vi "WS1050 36 DUT Characterization Ver1.1.vi"() -> ()   [LabVIEW 2012]
uses:
  WS_VCAP Driver 029/Source/WSVCAP Shell/Type Defs/WSVCAP SHL I2C DUT Mask Mode Enum.ctl
  <vilib>/Utility/file.llb/Read From Spreadsheet File (DBL).vi
panel:
  out "VISA resource name out":refnum<visa-resource-name>="GPIB0::3::INSTR"
  out "error out 2":errorcluster={"status"=TRUE, "code"=-63192, "source"="niLvFpga_Open_PXI-7813R.vi"}
  in  "Reg1_Bit Cntrl":string[](array[string])=["01", "02", "04", "08", "10", "20", "40", "80", "03", "06", "0C", "D8", "33", "66", "CC", "07", "0E", "1C", "38", "70", "E0", "0F", "1E", "3C", "78", "F0", "1F", "3E", "7C", "F8", "3F", "7E", "FC", "7F", "FE", "FD", "FB", "F7", "EF", "DF", "BF", "7F", "FC", "F9", "F3", "E7", "CF", "9F", "3F", "F8", "F1", "E3", "C7", "8F", "1F", "F0", "E1", "C3", "87", "0F", "E0", "C1", "83", "07", "C0", "81", "03", "AA", "55", "00"]
  out "date string":string="5/19/2014"
  out "PS1 Out":refnum<visa-resource-name>
  out "Ke2000 Out":refnum<visa-resource-name>="GPIB0::9::INSTR"
  in  "VPI_Cmd":string[](array[string])=["00", "3B", "00"]
  in  "VPI Name":string[](array[string])=["All_Drivers OFF", "All Drivers ON", "All Drivers OFF2"]
  in  "Tab Control":T1(tab)
  in  "No of Cmd":i64=3
  in  "Board#":string="BRD5"
  in  "Serial Number":string[][](table)=[["DUT", "SN"], ["DUT1", "1"], ["DUT2", "2"], ["DUT3", "3"], ["DUT4", "4"], ["DUT5", "5"], ["DUT6", "6"], ["DUT7", "7"], ["DUT8", "8"], ["DUT9", "9"], ["DUT10", "10"], ["DUT11", "11"], ["DUT12", "12"], ["DUT13", "13"], ["DUT14", "14"], ["DUT15", "15"], ["DUT16", "16"], ["DUT17", "17"], ["DUT18", "18"], ["DUT19", "19"], ["DUT20", "20"], ["DUT21", "21"], ["DUT22", "22"], ["DUT23", "23"], ["DUT24", "24"], ["DUT25", "25"], ["DUT26", "26"], ["DUT27", "27"], ["DUT28", "28"], ["DUT29", "29"], ["DUT30", "30"], ["DUT31", "31"], ["DUT32", "32"], ["DUT33", "33"], ["DUT34", "34"], ["DUT35", "35"], ["DUT36", "36"]]
  in  "SPI Clock Rate (Hz)":dbl=5000000.0 caption="Cycle Speed" format="%.1p Hz"
  in  "Wafer#":string="T7-EB"
  in  "File Name":string="CYC_WS1050_T7_EB_65C_40V_25DC_EMPTY_BRD5_141017_1"
  in  "TMN DC\\CAP Data Log File Path":path=path "C:/WS1050 36 DUT Data"
  in  "Test Program":string="WS1050 36 DUT Characterization Ver1.1"
  out "Current Date":string="8/28/2014"
  out "Current Time":string="0950"
  in  "Start Date":string="10/21/2014"
  in  "Start Time":string="1542"
  in  "Comment":string="CYC65C40V"
  in  "OK Button":bool
  in  "Calibration":bool
  in  "Verify CP":bool
  in  "CP Setting":i32(ring) items=["CP OFF", "CP ON", "CP 35V", "CP 40V", "DVA ON", "DVA OFF", "REG1 ON", "REG1 OFF", "REG2 ON", "REG2 OFF", "REG3 ON", "REG3 OFF"]
  in  "Stop Calibration":bool
  in  "Set VDD":dbl=3.7 format="%.3g"
  in  "Command":string[](array[string])=["07020100003B", "070201003B00", "0702013B0000"]
  in  "Clock Rate (Hz)":dbl=1000000.0 caption="Meas Speed" format="%.1p Hz"
  out "AR  Measurent(Hz)":dbl
  in  "PS1 Source":refnum<visa-resource-name>="GPIB0::5::INSTR"
  in  "Ke2000":refnum<visa-resource-name>="GPIB0::9::INSTR"
  in  "Set CP to Meas":i32(ring) items=["CP OFF", "CP 23.75V ", "CP 24.5V", "CP 25.25V", "CP 26V", "CP 26.75V", "CP 27.5V", "CP 28.25V", "CP 29V", "CP 29.75V", "CP 30.5V", "CP 31.25V", "CP 32V", "CP 32.75V", "CP 33.5V", "CP 34.25V", "CP 35V", "CP 35.75V", "CP 36.5V", "CP 37.25V", "CP 38V", "CP 38.75V", "CP 39.5V", "CP 40.25V", "CP 41V", "CP 41.75V", "CP 42.5V", "CP 43.25V", "CP 44V", "CP 50V", "CP 55V"]
  out "Simulate FPGA":bool
  out "Online":bool
  out "AR Cycling(Hz)":dbl=5000000.0
  in  "Ke2400":refnum<visa-resource-name>="GPIB0::3::INSTR"
  in  "Initialize AD7747":bool
  in  "DUT Mask Mode":T2=enum."All"
  in  "RFFE Slave Address":u8=7 caption="Slave Address" format="0x%02x"
  out "Activity Log":string="05/19/2014 -- 12:24:35.853::WSVCAP::APP::Application Started\n05/19/2014 -- 12:24:37.606::WSVCAP::WSVCAP SHL::WR I2C-REG:0x0A;MASK:0xFFFFFFFFFFFF;C1 DATA:22:22:22:22:22:22:22:22:22:22:22:22:22:22:22:22;C2 DATA:22:22:22:22:22:22:22:22:22:22:22:22:22:22:22:22;C3 DATA:22:22:22:22:22:22:22:22:22:22:22:22:22:22:22:22\r\n05/19/2014 -- 12:24:37.773::WSVCAP::WSVCAP SHL::WR I2C-ST:0,0,4,1\r\n05/19/2014 -- 12:24:37.903::WSVCAP::WSVCAP SHL::RD I2C-BYTES:4;ADD:0x00;MASK:0xFFFFFFFFFFFF\r\n05/19/2014 -- 12:24:38.045::WSVCAP::WSVCAP SHL::RD I2C:C1 DATA:2:2:2:2:2:2:2:2:2:2:2:2:2:2:2:2|A7:A9:AA:82:82:7F:82:81:82:81:83:82:81:82:82:81|46:36:BB:88:44:A3:E9:2B:32:20:ED:25:BB:3D:68:B|2C:6A:EB:A7:22:56:FE:CC:36:82:D7:B0:3B:48:F9:CC;C2 DATA:2:2:2:2:2:2:2:2:2:2:2:2:2:2:2:2|94:94:94:80:80:80:80:80:81:7E:7E:81:80:7E:80:80|47:33:15:82:62:B:E8:1C:D7:C3:7D:41:7C:B7:4C:2A|C4:B4:AE:8:1E:D1:4E:37:11:C0:6F:63:42:9D:63:B5;C3 DATA:2:2:2:2:2:2:2:2:2:2:2:2:2:2:2:2|95:95:95:81:81:7E:81:80:84:7D:80:83:81:7E:7F:80|AB:C4:14:B5:7B:52:DF:C9:79:5D:5F:30:99:31:1E:F4|6E:5C:F7:A8:C3:EB:7B:EF:33:92:89:77:4D:67:75:DD;STATUS:0:0:4:0\r\n05/19/2014 -- 12:24:38.046::WSVCAP::WSVCAP SHL::WR I2C-REG:0x0A;MASK:0xFFFFFFFFFFFF;C1 DATA:22:22:22:22:22:22:22:22:22:22:22:22:22:22:22:22;C2 DATA:22:22:22:22:22:22:22:22:22:22:22:22:22:22:22:22;C3 DATA:22:22:22:22:22:22:22:22:22:22:22:22:22:22:22:22\r\n05/19/2014 -- 12:24:38.089::WSVCAP::WSVCAP SHL::WR I2C-ST:0,0,4,1\r\n05/19/2014 -- 12:24:38.219::WSVCAP::WSVCAP SHL::RD I2C-BYTES:4;ADD:0x00;MASK:0xFFFFFFFFFFFF\r\n05/19/2014 -- 12:24:38.362::WSVCAP::WSVCAP SHL::RD I2C:C1 DATA:2:2:2:2:2:2:2:2:2:2:2:2:2:2:2:2|A7:AB:AA:82:82:82:83:83:82:82:82:82:7F:82:82:81|4B:32:96:83:3E:61:43:17:25:62:AB:4D:A2:40:2E:5|3C:76:2B:B4:EE:E4:A9:1A:AA:A:26:C7:21:2E:87:5B;C2 DATA:2:2:2:2:2:2:2:2:2:2:2:2:2:2:2:2|94:94:94:80:80:80:80:80:80:7F:80:81:80:80:7F:80|4A:32:19:7D:19:6C:79:46:61:7F:4B:B8:A5:30:F3:14|B4:70:A:8C:9C:DC:43:FA:1E:A:C6:21:A:A9:13:F3;C3 DATA:2:2:2:2:2:2:2:2:2:2:2:2:2:2:2:2|95:97:94:81:80:81:82:81:80:7E:81:84:7F:81:80:80|B2:32:D0:A7:9E:4C:AB:D4:EE:D9:F0:82:B7:91:7:FF|C1:91:B6:3D:D8:E:1B:4F:9F:6A:F1:6C:E7:3F:7:BA;STATUS:0:0:4:0\r\n05/19/2014 -- 12:24:38.364::WSVCAP::WSVCAP SHL::WR I2C-REG:0x0A;MASK:0xFFFFFFFFFFFF;C1 DATA:22:22:22:22:22:22:22:22:22:22:22:22:22:22:22:22;C2 DATA:22:22:22:22:22:22:22:22:22:22:22:22:22:22:22:22;C3 DATA:22:22:22:22:22:22:22:22:22:22:22:22:22:22:22:22\r\n05/19/2014 -- 12:24:38.406::WSVCAP::WSVCAP SHL::WR I2C-ST:0,0,4,1\r\n05/19/2014 -- 12:24:38.536::WSVCAP::WSVCAP SHL::RD I2C-BYTES:4;ADD:0x00;MASK:0xFFFFFFFFFFFF\r\n05/19/2014 -- 12:24:38.678::WSVCAP::WSVCAP SHL::RD I2C:C1 DATA:2:2:2:2:2:2:2:2:2:2:2:2:2:2:2:2|A7:A9:AB:82:82:81:82:82:82:82:82:82:82:82:82:81|46:71:4C:87:43:3D:7F:FC:25:4F:8E:54:97:3E:60:8C|AA:F4:1F:B5:CE:43:1F:36:9:87:9C:78:86:5:B6:8E;C2 DATA:2:2:2:2:2:2:2:2:2:2:2:2:2:2:2:2|94:94:94:80:7F:7F:80:80:80:80:80:81:80:80:80:80|49:36:18:7D:6E:C5:E4:3C:81:2E:41:D3:75:71:E3:72|E8:D3:E6:D1:E0:48:AE:D4:54:D:E8:8E:B4:41:68:4;C3 DATA:2:2:2:2:2:2:2:2:2:2:2:2:2:2:2:2|95:95:95:81:7F:7F:81:81:81:81:81:84:81:81:82:81|B3:F5:90:AB:82:69:7B:93:D0:77:E8:D5:E8:8C:84:E8|B9:AC:EE:2B:B6:71:8F:4A:74:31:56:BB:8A:B7:A0:C8;STATUS:0:0:4:0\r\n05/19/2014 -- 12:24:38.681::WSVCAP::WSVCAP SHL::WR I2C-REG:0x0A;MASK:0xFFFFFFFFFFFF;C1 DATA:22:22:22:22:22:22:22:22:22:22:22:22:22:22:22:22;C2 DATA:22:22:22:22:22:22:22:22:22:22:22:22:22:22:22:22;C3 DATA:22:22:22:22:22:22:22:22:22:22:22:22:22:22:22:22\r\n05/19/2014 -- 12:24:38.723::WSVCAP::WSVCAP SHL::WR I2C-ST:0,0,4,1\r\n05/19/2014 -- 12:24:38.854::WSVCAP::WSVCAP SHL::RD I2C-BYTES:4;ADD:0x00;MASK:0xFFFFFFFFFFFF\r\n05/19/2014 -- 12:24:38.996::WSVCAP::WSVCAP SHL::RD I2C:C1 DATA:2:2:2:2:2:2:2:2:2:2:2:2:2:2:2:2|A7:A9:AA:82:82:7F:83:81:82:81:84:82:7F:82:7F:82|43:FB:E:7F:3C:AD:35:35:26:A2:6C:21:4B:3D:8:6|63:9A:E1:F3:95:32:91:42:90:3C:78:1F:5C:D7:5F:D8;C2 DATA:2:2:2:2:2:2:2:2:2:2:2:2:2:2:2:2|94:94:94:80:80:80:80:80:81:80:7E:81:80:7E:7F:80|48:36:18:7F:5E:3D:69:83:DE:AE:A1:9E:31:AE:BB:96|15:A0:44:17:13:FD:CC:C8:6D:B2:EF:A7:C:C7:3B:F;C3 DATA:2:2:2:2:2:2:2:2:2:2:2:2:2:2:2:2|95:96:94:81:81:7E:82:80:84:80:80:84:7F:7E:7D:82|AD:3B:6D:A9:7C:57:9D:F5:7A:96:23:5C:36:2D:ED:5A|CD:46:DB:3B:C7:BD:70:60:33:B8:B:F7:63:A:51:4D;STATUS:0:0:4:0\r\n05/19/2014 -- 12:24:38.998::WSVCAP::WSVCAP SHL::WR I2C-REG:0x0A;MASK:0xFFFFFFFFFFFF;C1 DATA:22:22:22:22:22:22:22:22:22:22:22:22:22:22:22:22;C2 DATA:22:22:22:22:22:22:22:22:22:22:22:22:22:22:22:22;C3 DATA:22:22:22:22:22:22:22:22:22:22:22:22:22:22:22:22\r\n05/19/2014 -- 12:24:39.040::WSVCAP::WSVCAP SHL::WR I2C-ST:0,0,4,1\r\n05/19/2014 -- 12:24:39.170::WSVCAP::WSVCAP SHL::RD I2C-BYTES:4;ADD:0x00;MASK:0xFFFFFFFFFFFF\r\n05/19/2014 -- 12:24:39.311::WSVCAP::WSVCAP SHL::RD I2C:C1 DATA:2:2:2:2:2:2:2:2:2:2:2:2:2:2:2:2|A7:AA:AB:82:82:81:82:81:82:81:82:82:82:82:7F:82|44:F1:90:87:45:44:C8:2C:2C:F1:FC:1B:94:3B:3C:75|4A:49:95:19:99:73:64:3:23:24:F3:A2:5E:7F:C4:B6;C2 DATA:2:2:2:2:2:2:2:2:2:2:2:2:2:2:2:2|94:94:94:80:80:80:80:7F:80:80:7E:80:80:7E:7F:80|4C:36:17:7D:A8:9F:DE:C7:53:6D:8A:F4:41:A5:C6:E0|90:2E:24:C:D9:22:E4:76:3B:40:1D:53:33:B1:3E:4D;C3 DATA:2:2:2:2:2:2:2:2:2:2:2:2:2:2:2:2|95:97:95:81:81:7F:81:80:80:81:7F:82:81:7E:7D:82|AE:2B:A7:AB:CC:CD:A4:38:FD:17:80:F2:92:2D:45:C4|76:E5:D:B9:AD:B5:BA:8D:28:32:9E:42:B7:20:4A:D9;STATUS:0:0:4:0\r\n05/19/2014 -- 12:24:39.313::WSVCAP::WSVCAP SHL::WR I2C-REG:0x0A;MASK:0xFFFFFFFFFFFF;C1 DATA:22:22:22:22:22:22:22:22:22:22:22:22:22:22:22:22;C2 DATA:22:22:22:22:22:22:22:22:22:22:22:22:22:22:22:22;C3 DATA:22:22:22:22:22:22:22:22:22:22:22:22:22:22:22:22\r\n05/19/2014 -- 12:24:39.355::WSVCAP::WSVCAP SHL::WR I2C-ST:0,0,4,1\r\n05/19/2014 -- 12:24:39.486::WSVCAP::WSVCAP SHL::RD I2C-BYTES:4;ADD:0x00;MASK:0xFFFFFFFFFFFF\r\n05/19/2014 -- 12:24:39.628::WSVCAP::WSVCAP SHL::RD I2C:C1 DATA:2:2:2:2:2:2:2:2:2:2:2:2:2:2:2:2|A7:A9:AA:82:82:82:83:82:82:82:82:82:7F:82:7F:82|47:18:E4:87:3E:E7:6:65:25:92:37:38:A8:3E:89:85|7C:A7:7:2B:A3:7A:EC:EF:89:ED:F4:D3:D8:BC:3A:F5;C2 DATA:2:2:2:2:2:2:2:2:2:2:2:2:2:2:2:2|94:94:94:80:7F:80:80:7F:81:80:7E:80:80:80:81:80|49:37:17:80:76:25:6A:F8:DF:55:97:4D:B8:5B:2B:B1|13:E3:9A:3E:1A:2D:4F:B6:DB:E9:61:FA:8B:D6:9:CC;C3 DATA:2:2:2:2:2:2:2:2:2:2:2:2:2:2:2:2|95:95:95:81:7F:80:82:81:84:80:7F:81:80:81:7F:82|AF:93:3B:AF:5B:11:82:E4:7E:C3:2D:72:9:96:D9:A|DB:96:F2:10:5F:64:9A:C6:98:12:27:7D:10:D3:20:D9;STATUS:0:0:4:0\r\n05/19/2014 -- 12:24:40.132::WSVCAP::WSVCAP SHL::CLOSE\r\n"
  in  "C1 Cap DAC":u8=128 caption="B Data In" format="0x%02x"
  in  "C2 Cap DAC":u8=128 caption="B Data In" format="0x%02x"
  in  "C3 Cap DAC":u8=128 caption="B Data In" format="0x%02x"
  out "IDD Brd(uA)":string
  in  "CP to Meas":i32(ring)=1 items=["CP HDC 35V", "CP HDC 40.25V", "CP HDC 27.5V", "CP HDC 30.5V", "CP HDC 44V"]
  in  "CP VPI":i32(ring) items=["CP HDC 35V", "CP HDC 40.25V", "CP HDC 27.5V", "CP HDC 30.5V", "CP HDC 44V"]
  in  "Repeat Meas(s)":u32
  in  "Real No. From\nLookup Table":bool
  in  "Control Panel":T3={"CP C-V \nSweep"=TRUE, "HD/CYC"=FALSE, "E-CAL"=FALSE, "DVA"=FALSE, "VPI"=FALSE, "VSA"=FALSE, "HS"=FALSE}
  out "CP C-V Sweep":bool
  out "HD/CYC":bool
  out "E-CAL":bool
  out "DVA":bool
  out "VPI":bool
  out "VSA":bool
  out "HS":bool
  in  "Lot#":string="WS1050"
  out "AD7747 Values":string[][](table)
  in  "Freq(Hz)":string="12K"
  in  "Reset P/S":bool
  in  "Test Sequences":i32(ring) items=["C1_C2_C3", "C2_C1_C3", "C3_C2_C1"]
  in  "WS1050/51":bool=TRUE
  in  "CP with DVA ON":i32(ring) items=["CP HDC 35V", "CP HDC 40.25V", "CP HDC 27.5V", "CP HDC 30.5V", "CP HDC 44V"]
  in  "% Duty Cycle":string="NA"
  in  "Cmd To HD":string="0702013B3B3B"
  in  "Post CMd Delay":dbl[](array[numeric])=[1.8e-05, 1.8e-05, 1.8e-05] min=0.0 max=0.5 format="%#.0p s"
  in  "Cmin/Act":bool=TRUE
  out "40V_1":string[][](table)
  out "NOM IDD OFF(uA)":string
  out "40V_2":string[][](table)
  out "40V_3":string[][](table)
  out "Total Time":u64
  in  "Set HD/Cycle \nto Complete":u64=50000000000
  out "No of HD/Cycle\nCompleted":u64
  out "Cycle Count":u64 min=1 max=4 step=1
  out "Loop \ncompleted":i32=1
  out "Previous Time":string="12:20:26 PM"
  out "STATUS":string="Idle...."
  out "Total Delta C2(pF)":string[](array[string])
  out "Total Delta C1(pF)":string[](array[string])
  out "Total Delta C3(pF)":string[](array[string])
  out "RB Reg for HD":string[](array[string])
  out "RB Reg for HD/Cycle":string[](array[string])
  out "VPI C2":string[][](table)
  out "VPI C3":string[][](table)
  out "NOM IDD ON (uA)":string
  out "IDD_HD/CYC (uA)":string="164.601255E+0"
  in  "stop During HD/Cycles":bool
  in  "stop":bool
  out "IDD Stdby(uA)":string="2.606990E+0"
  out "VPI C1":string[][](table)
  out "Loops Run":u64
  out "CP Voltage":string
  out "VSA_V1":string[][](table)
  out "VSA_V2":string[][](table)
  out "VSA_V3":string[][](table)
  in  "VSA Voltage(V)":dbl[](array[numeric])=[-10.0, 0.0, 10.0]
  in  "DC_Temp":i32=25
  in  "HD/CYC Temp":i32=25
  in  "Time All ON (s)":u32=120
  in  "Time All OFF (s)":u32=120
  in  "HD_DC (Min)":u64=259200
  out "LPs Count":i32
  in  "X Repeat":i32=100
  out "No LPs to RP":i32
  out "Run Loops":i32=1
  out "TTCompleted":u64=2000
  in  "TTF Completed":u64=50000000000
  out "% Delta C_T0":string[][](array[string])
  out "% Delta C":string[][](array[string])
  out "EFuse RB T0":string[](array[string])
  out "Current EFuse Read back":string[](array[string])
  out "EFuse Readback Status":bool[](array[boolean])
  in  "DeltaC Target Setting(pF)":dbl=7.375
  out "error out":errorcluster
  in  "error in (no error)":errorcluster
  in  "HD RP":dbl=60.0
  in  "Cycle RP":dbl=10000.0
  out "Plot_1":dbl[][](graph) caption="(Y) Multi Plot 2"
  out "Plot_2":dbl[][](graph) caption="(Y) Multi Plot 2"
  out "Plot_3":dbl[][](graph) caption="(Y) Multi Plot 2"
  in  "Debug":bool
  in  "No of Rows\nFrom Spread Sheet":i32
  in  "Plot Delta Cmin":bool=TRUE
  in  "Plot":T4(ring)
  in  "Bank 2":i32(ring)=4 items=["C1", "C2", "C3", "D_C1", "D_C2", "D_C3"]
  in  "Bank":i32(ring)=3 items=["C1", "C2", "C3", "D_C1", "D_C2", "D_C3"]
  in  "Bank 3":i32(ring)=5 items=["C1", "C2", "C3", "D_C1", "D_C2", "D_C3"]
  # "Company:  WiSpry Inc\n20 Fairbanks Ste 198 Irvine CA 92618\n\nAuthor:  Andy V Tran\nCreated:  07/15/2015\nLabVIEW 2012 Pro\nTest Program:  WS1050 36 DUT Characterization Ver1.1\nFPGA: WS_VCAP Driver 029"
  # "Note for HD Duty Cycle:\n1.  Set time to start HD_DC (Min), default is 259200 (6 months) \n2.  Set Time for Duty Cycle ON/OFF, default setting is 2 minutes\n3.  No of Loops to RP = 3600s/(Time ALL ON(s) + Time ALL + OFF(s))\n4.  Set X Repeat = no of runs, default is 100 runs\n5.  Set TTF Completed to stop the test.\n\nVer 1.1 updated based on Ver1.0:\n1.  Updated the control panel ( CP C-V Sweep was set \"Yes\" by default)\n2.  CP Voltage sweep should be set up from look up table."
  # "Minutes"
  # "X1000"
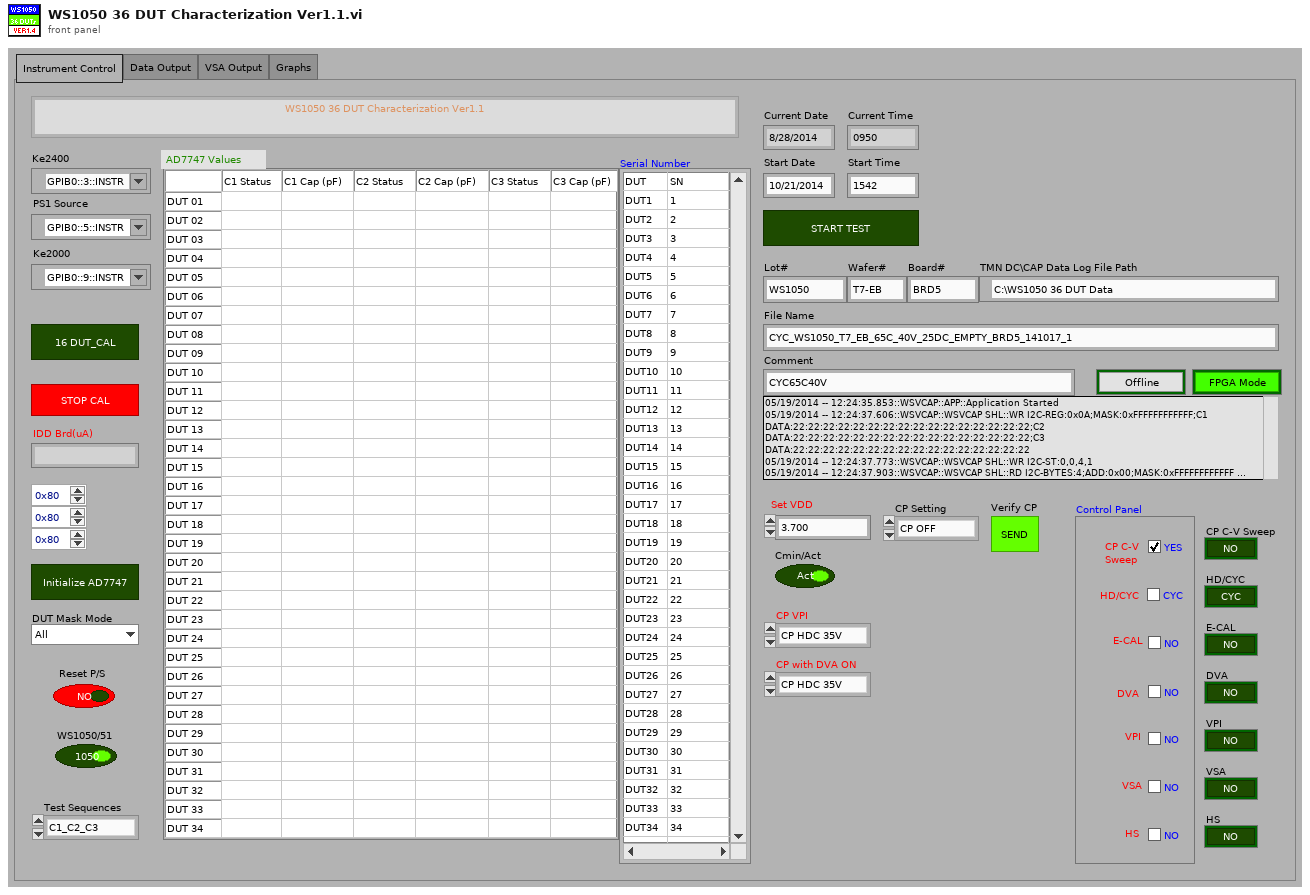
[diagram p1: front panel]
types:
  T1 = enum32{"Instrument Control", "Data Output", "VSA Output", "Graphs"}
  T2 = typedef "WSVCAP SHL I2C DUT Mask Mode Enum.ctl" = enum16{"Custom", "C1", "C2", "C3", "All"}
  T3 = cluster{"CP C-V \nSweep":bool, "HD/CYC":bool, "E-CAL":bool, "DVA":bool, "VPI":bool, "VSA":bool, "HS":bool}
  T4 = enum16{"ALL DUTs", "DUT 01", "DUT 02", "DUT 03", "DUT 04", "DUT 05", "DUT 06", "DUT 07", "DUT 08", "DUT 09", "DUT 10", "DUT 11", "DUT 12", "DUT 13", "DUT 14", "DUT 15", "DUT 16", "DUT 17", "DUT 18", "DUT 19", "DUT 20", "DUT 21", "DUT 22", "DUT 23", "DUT 24", "DUT 25", "DUT 26", "DUT 27", "DUT 28", "DUT 29", "DUT 30", "DUT 31", "DUT 32", "DUT 33", "DUT 34", "DUT 35", "DUT 36"}
  T5 = typedef "WSVCAP SHL Core System Cluster.ctl" = cluster{"Settings":T6, "FPGA Resource":tag, "Online":bool, "I2C Wait Ticks":u32, "SPI Wait Ticks":u32, "RFFE Wait Ticks":u32}
  T6 = typedef "WSVCAP SHL I2C Settings Cluster.ctl" = cluster{"FPGA Resource Name":string, "I2C Slave Address":u8, "I2C Clock Rate (Hz)":dbl, "SPI Clock Rate (Hz)":dbl, "RFFE Slave Address":u8, "RFFE Clock Rate (Hz)":dbl, "Simulate FPGA":bool, "C1 Cap DAC Default":u8, "C2 Cap DAC Default":u8, "C3 Cap DAC Default":u8}
  T7 = enum16{"Idle...", "Voltage 1", "Voltage 2", "Voltage 3"}[]
  T8 = cluster{"Test Program ":string, "Comment":string, "Data Out":string, "Data Out":string, "CP Voltage":string, string, "Data Out":string, "CP Voltage":string, "string":string, "Freq(Hz)":string, "Board#":string}
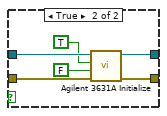
[diagram p2: hidden frame]
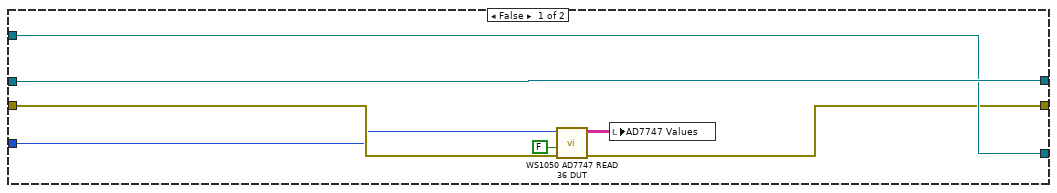
[diagram p10: hidden frame]
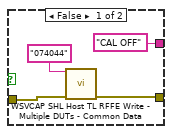
[diagram p11: hidden frame]
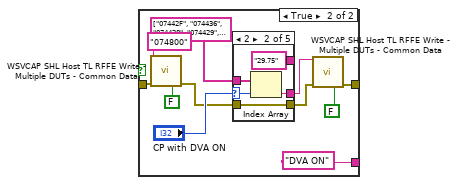
[diagram p12: hidden frame]
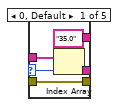
[diagram p13: hidden frame]
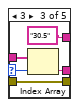
[diagram p14: hidden frame]
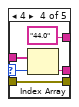
[diagram p15: hidden frame]
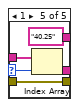
[diagram p16: hidden frame]
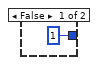
[diagram p17: hidden frame]
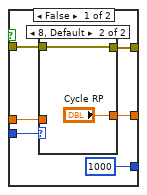
[diagram p18: hidden frame]
diagram:
  w19 = TRUE
  w25 = u16 0 items=["Off", "Moving Filter", "Repeating Filter"] ("Digital Filter (0: Off)")
  w26 = u16 7 items=["3.5 Digits"=4, "4.5 Digits"=5, "5.5 Digits"=6, "6.5 Digits"=7] ("Resolution (7: 6.5 digits)")
  n1 = case shown="True" w19 {
    tunnel: "error in (no error)" -> [w33 w34]
    tunnel: [w33 w41] -> w5
    frame False {
    }
    frame True {
      n2 = call "WSVCAP SHL Host TL Initialize.vi"("error in"=w34) -> ("error out"=w35:errorcluster)  [unwired: 13 in, 1 out]
      n3 = control-ref of="Activity Log"() -> (w37:refnum<vi>)
      n4 = call "ACT LG Activity Log Core.vi"("Display Ref"=w37, "Source"="WSVCAP", "Error In (no error)"=w35) -> ("Error Out"=w36:errorcluster)  [unwired: 11 in, 1 out]
      n5 = call "WSVCAP SHL Host TL Status Manager.vi"("error in"=w36) -> ("System Out"=w42:T5, "error out"=w41:errorcluster)  [unwired: 13 in]
      n6 = Unbundle By Name(w42) -> ("Online"=→"Online":bool, "Settings.Simulate FPGA"=→"Simulate FPGA":bool)
    }
  }
  n7 = case shown="True" TRUE {
    tunnel: w5 -> [w43 w48]
    tunnel: [w44 w47] -> w16
    tunnel: [w43 w46] -> w9
    tunnel: "Ke2400" -> [w44 w45]
    frame False {
    }
    frame True {
      n8 = VISA Write(VISA resource name=w45, write buffer="SOUR:FUNC VOLT;VOLT:MODE FIX;RANG 100;LEV 0.0;:SENS:FUNC \"CURR\";CURR:PROT 60E-3;RANG 100E-3;:OUTP ON", error in (no error)=w48) -> (VISA resource name out=w47:refnum<visa-resource-name>, error out=w46:errorcluster)  [unwired: 1 out]
    }
  }
  n9 = case shown="False" "Reset P/S" {
    tunnel: "PS1 Source" -> [w50 w57]
    tunnel: [w50 w55] -> w30
    tunnel: w5 -> [w51 w53]
    tunnel: [w51 w52] -> w4
    frame False {
    }
    frame True {
      n10 = call "Agilent 3631A Initialize.vi"("error in (no error)"=w53, "Default"=FALSE ("Reset? (T: Yes)"), "Reset"=TRUE ("ID Query? (T: Yes)"), "VISA resource name"=w57) -> ("error out"=w52:errorcluster, "VISA resource name out"=w55:refnum<visa-resource-name>)  [unwired: 6 in]
    }
  }
  n11 = call "Ke2000 Initialize.vi"("error in (no error)"=w5, "VISA resource name"="Ke2000") -> ("error out"=w27:errorcluster, "VISA resource name out"=w28:refnum<visa-resource-name>)  [unwired: 8 in]
  n12 = call "Ke2000 Configure DC Current.vi"("Resolution (7: 6.5 digits)"=w26, "Digital Filter (0: Off)"=w25, "Auto Range? (T: Auto)"=FALSE, "error in (no error)"=w27, "Custom Range (0 A)"=1.0, "VISA resource name"=w28) -> ("error out"=w6:errorcluster, "VISA resource name out"=w23:refnum<visa-resource-name>)  [unwired: 4 in]
  n13 = case shown="True" TRUE {
    tunnel: [_ w58] -> w32
    frame False {
    }
    frame True {
      n14 = call-poly <vilib>:"Read From Spreadsheet File.vi"("number of rows (all:-1)"=-1) -> ("all rows"=w58:dbl[][])  [unwired: 6 in, 4 out]
    }
  }
  n15 = Merge Errors(w9, w6, w4) -> (w17:errorcluster)
  n16 = while {
    tunnel: w17 -> [w62]
    tunnel: [w71] -> w13
    tunnel: w32 -> [w87]
    tunnel: w30 -> [w75]
    tunnel: w23 -> [w76]
    tunnel: [w85] -> w22
    tunnel: [w84] -> w21
    tunnel: w16 -> [w82]
    tunnel: [w81] -> w14
    tunnel: [FALSE ("stop")] -> w7
    i -> [w83]
    stop <- w88 stop-if-true
    n17 = case shown="0" w83 {
      tunnel: w62 -> [w99 w101]
      tunnel: [w98 w101] -> w78
      tunnel: "RFFE Slave Address" -> [w96 _]
      frame 0 {
        w92 = dbl[][] []
        w91 = "" ("uA")
        w93 = string[][] []
        w94 = string[] [] ("EFuse Read back")
        w100 = u64 0 ("No of HD/Cycle\nCompleted")
        n18 = local write "RB Reg for HD/Cycle"(w94) -> ()
        n19 = local write "Current EFuse Read back"(w94) -> ()
        n20 = local write "EFuse RB T0"(w94) -> ()
        n21 = local write "Total Delta C1(pF)"(w94) -> ()
        n22 = local write "Total Delta C2(pF)"(w94) -> ()
        n23 = local write "Total Delta C3(pF)"(w94) -> ()
        n24 = local write "Cycle Count"(w100) -> ()
        n25 = local write "No of HD/Cycle\nCompleted"(w100) -> ()
        n26 = local write "NOM IDD OFF(uA)"(w91) -> ()
        n27 = local write "NOM IDD ON (uA)"(w91) -> ()
        n28 = local write "IDD Brd(uA)"(w91) -> ()
        n29 = local write "40V_2"(w93) -> ()
        n30 = local write "VPI C2"(w93) -> ()
        n31 = local write "VSA_V2"(w93) -> ()
        n32 = local write "VPI C1"(w93) -> ()
        n33 = local write "VPI C3"(w93) -> ()
        n34 = local write "% Delta C_T0"(w93) -> ()
        n35 = local write "40V_1"(w93) -> ()
        n36 = local write "VSA_V3"(w93) -> ()
        n37 = local write "40V_3"(w93) -> ()
        n38 = local write "VSA_V1"(w93) -> ()
        n39 = local write "% Delta C"(w93) -> ()
        n40 = call "WSVCAP SHL Host TL RFFE Configure.vi"("RFFE Slave Address"=w96, "Clock Rate (Hz)"="Clock Rate (Hz)", "error in"=w99) -> ("Actual Rate (Hz)"=→"AR  Measurent(Hz)":dbl, "error out"=w98:errorcluster)  [unwired: 11 in]
        n41 = local write "Plot_3"(w92) -> ()
        n42 = local write "Plot_2"(w92) -> ()
        n43 = local write "Plot_1"(w92) -> ()
      }
      frame 1, Default {
      }
    }
    n44 = while {
      tunnel: ["stop"] -> w80
      tunnel: w78 -> [w127]
      tunnel: [w119] -> w72
      tunnel: w75 -> [w126]
      tunnel: w76 -> [w121]
      tunnel: [w122] -> w74
      tunnel: [w120] -> w73
      tunnel: [w117] -> w69
      tunnel: [w116] -> w68
      tunnel: [w115] -> w67
      tunnel: [w114] -> w66
      tunnel: [w113] -> w65
      tunnel: [w112] -> w64
      tunnel: [w111] -> w63
      tunnel: ["Command"] -> w61
      tunnel: ["Post CMd Delay"] -> w60
      stop <- w134 stop-if-true
      # "Set Date & Time to Start Test"
      n45 = case shown="True" "Initialize AD7747" {
        tunnel: w127 -> [w143 w148]
        tunnel: [w143 w144] -> w110
        tunnel: w126 -> [w142 w146]
        tunnel: [w142 w145] -> w125
        frame False {
        }
        frame True {
          w149 = T7 [enum."Voltage 2", enum."Voltage 3", enum."Voltage 1"] items=["Idle...", "Voltage 1", "Voltage 2", "Voltage 3"]
          n46 = for {
            tunnel: w146 -> [w159]
            tunnel: w149 -> [w157] mode=indexing
            tunnel: [w156] -> w145
            shift-right: [w152] -> w147
            shift-left: w148 -> [w160]
            n47 = local read "Set VDD"() -> (w155:dbl)
            n48 = call "E3631A_Voltage Controller updated.vi"("VISA resource name"=w159, "I_VDD(A)"=0.5, "Channel Controller"=w157, "Voltage 1"=w155, "Voltage 2"=3.3, "error in (no error)"=w160, "I_3.3V (A)"=0.5) -> ("VISA resource name out"=w156:refnum<visa-resource-name>, "error out"=w151:errorcluster)  [unwired: 7 in]
            n49 = call "Delay T4.vi"("milliseconds to wait"=u32 100, "error in (no error)"=w151) -> ("error out"=w152:errorcluster)  [unwired: 9 in]
          }
          n50 = call "WS1050_AD7747_Init 36DUT.vi"("error in"=w147) -> ("error out"=w144:errorcluster)  [unwired: 10 in]
        }
      }
      n51 = call "Time_stamp.vi"() -> ("date/time string"=w139:string, "date string"=w141:string)  [unwired: 2 in]
      "Current Date" <- w141
      "Current Time" <- w139
      n52 = Equal?(x=w141, y="Start Date") -> (x = y?=w137:bool)
      n53 = Equal?(x=w139, y="Start Time") -> (x = y?=w136:bool)
      n54 = And(x=w137, y=w136) -> (x .and. y?=w133:bool)
      n55 = Compound Arithmetic op=OR(w133, "OK Button", "stop") -> (w134:bool)
      n56 = case shown="True" "Calibration" {
        tunnel: w110 -> [w190 w204]
        tunnel: [w184 w201] -> w108
        tunnel: w125 -> [w189 w200]
        tunnel: "DUT Mask Mode" -> [w188 w196]
        tunnel: [w189 w195] -> w123
        tunnel: w121 -> [w187 w194]
        tunnel: [w187 w191] -> w120
        frame False {
          n57 = call "WS1050 AD7747 READ 36 DUT.vi"("error in"=w190, "Log (T)"=FALSE, "DUT Mask Mode (All)"=w188) -> ("error out"=w184:errorcluster, "AD7747 Values"=w185:string[][])  [unwired: 7 in]
          n58 = local write "AD7747 Values"(w185) -> ()
        }
        frame True {
          n59 = flat-sequence {
            tunnel: w204 -> [w213]
            tunnel: [w208] -> w203
            tunnel: w200 -> [w212]
            tunnel: [w211] -> w199
            tunnel: w196 -> [w210]
            tunnel: [w210] -> w197
            tunnel: w194 -> [w206]
            tunnel: [w205] -> w193
            tunnel: w203 -> [w236]
            tunnel: [w235] -> w202
            tunnel: w199 -> [w234]
            tunnel: [w234] -> w198
            tunnel: w197 -> [w233]
            tunnel: w193 -> [w229]
            tunnel: [w229] -> w192
            tunnel: w202 -> [w245]
            tunnel: [w248] -> w201
            tunnel: w198 -> [w247]
            tunnel: [w244] -> w195
            tunnel: w192 -> [w243]
            tunnel: [w243] -> w191
            frame #0 {
              w214 = T7 [enum."Voltage 2", enum."Voltage 3", enum."Voltage 1"] items=["Idle...", "Voltage 1", "Voltage 2", "Voltage 3"]
              n60 = for {
                tunnel: w212 -> [w224]
                tunnel: w214 -> [w222] mode=indexing
                tunnel: [w221] -> w211
                shift-right: [w219] -> w207
                shift-left: w213 -> [w225]
                w216 = 0.5 ("I_VDD(A)")
                n61 = local read "Set VDD"() -> (w217:dbl)
                n62 = call "E3631A_Voltage Controller updated.vi"("VISA resource name"=w224, "I_VDD(A)"=w216, "Channel Controller"=w222, "Voltage 1"=w217, "Voltage 2"=3.3, "error in (no error)"=w225, "I_3.3V (A)"=w216) -> ("VISA resource name out"=w221:refnum<visa-resource-name>, "error out"=w218:errorcluster)  [unwired: 7 in]
                n63 = call "Delay T4.vi"("milliseconds to wait"=u32 100, "error in (no error)"=w218) -> ("error out"=w219:errorcluster)  [unwired: 9 in]
              }
              n64 = call "Ke2000 Single Reading.vi"("error in (no error)"=w207, "VISA resource name"=w206) -> ("error out"=w208:errorcluster, "VISA resource name out"=w205:refnum<visa-resource-name>, "uA"=→"IDD Brd(uA)":string)  [unwired: 5 in, 2 out]
              n65 = One Button Dialog(message="Please verify all sockets should be empty...") -> ()  [unwired: 1 in, 1 out]
            }
            frame #1 {
              n66 = call "WS1050 CAPDAC Setting.vi"("DUT Mask Mode (All)"=w233, "error in"=w236, "C3 Cap DAC"="C3 Cap DAC", "C2 Cap DAC"="C2 Cap DAC", "C1 Cap DAC"="C1 Cap DAC") -> ("error out"=w231:errorcluster)  [unwired: 5 in, 1 out]
              n67 = call "WS1050 OFFSET CAL.vi"("error in"=w231, "OFFSET CAL"=TRUE ("Read?")) -> ("error out"=w230:errorcluster)  [unwired: 8 in, 1 out]
              n68 = while {
                tunnel: w230 -> [w242]
                tunnel: [w241] -> w235
                tunnel: w233 -> [w239]
                stop <- "Stop Calibration" stop-if-true
                n69 = call "WS1050 AD7747 READ 36 DUT.vi"("error in"=w242, "Log (T)"=FALSE, "DUT Mask Mode (All)"=w239) -> ("error out"=w241:errorcluster, "AD7747 Values"=→"AD7747 Values":string[][])  [unwired: 7 in]
              }
            }
            frame #2 {
              w246 = T7 [enum."Voltage 2", enum."Voltage 3", enum."Voltage 1"] items=["Idle...", "Voltage 1", "Voltage 2", "Voltage 3"]
              n70 = for {
                tunnel: w247 -> [w260]
                tunnel: w246 -> [w257] mode=indexing
                tunnel: [w256] -> w244
                shift-right: [w252] -> w248
                shift-left: w245 -> [w258]
                n71 = call "E3631A_Voltage Controller updated.vi"("VISA resource name"=w260, "I_VDD(A)"=0.5, "Channel Controller"=w257, "Voltage 1"=0.0, "Voltage 2"=3.3, "error in (no error)"=w258, "I_3.3V (A)"=0.5) -> ("VISA resource name out"=w256:refnum<visa-resource-name>, "error out"=w251:errorcluster)  [unwired: 7 in]
                n72 = call "Delay T4.vi"("milliseconds to wait"=u32 100, "error in (no error)"=w251) -> ("error out"=w252:errorcluster)  [unwired: 9 in]
              }
              n73 = One Button Dialog(message="Calibration Completed....") -> ()  [unwired: 1 in, 1 out]
            }
          }
        }
      }
      n74 = call "Control Panel.vi"("error in (no error)"=w110, "Control Panel"="Control Panel") -> ("error out"=w107:errorcluster, "VPI"=w113:bool, "DVA"=w114:bool, "E-CAL"=w115:bool, "VSA"=w112:bool, "HD/CYC"=w116:bool, "HS"=w111:bool, "Verify Socket"=w117:bool)  [unwired: 2 in]
      "CP C-V Sweep" <- w117
      "E-CAL" <- w115
      "VPI" <- w113
      "VSA" <- w112
      "HS" <- w111
      "HD/CYC" <- w116
      "DVA" <- w114
      n75 = Merge Errors(w107, w108) -> (w109:errorcluster)
      n76 = case shown="True" "Verify CP" {
        tunnel: [w161 w165] -> w119
        tunnel: w123 -> [w162 w168]
        tunnel: [w162 w166] -> w122
        tunnel: w109 -> [w161 w164]
        frame False {
        }
        frame True {
          w169 = T7 [enum."Voltage 2", enum."Voltage 3", enum."Voltage 1"] items=["Idle...", "Voltage 1", "Voltage 2", "Voltage 3"]
          # "Verify CP"
          n77 = for {
            tunnel: w168 -> [w182]
            tunnel: w169 -> [w180] mode=indexing
            shift-right: [w177] -> w167
            shift-left: w164 -> [w183]
            tunnel: [w175] -> w166
            n78 = local read "Set VDD"() -> (w179:dbl)
            n79 = call "E3631A_Voltage Controller updated.vi"("VISA resource name"=w182, "I_VDD(A)"=0.5, "Channel Controller"=w180, "Voltage 1"=w179, "Voltage 2"=3.3, "error in (no error)"=w183, "I_3.3V (A)"=0.5) -> ("VISA resource name out"=w175:refnum<visa-resource-name>, "error out"=w178:errorcluster)  [unwired: 7 in]
            n80 = call "Delay T4.vi"("milliseconds to wait"=u32 100, "error in (no error)"=w178) -> ("error out"=w177:errorcluster)  [unwired: 9 in]
          }
          n81 = Index Array(array=string[] ["074000", "074040", "07476F", "074776", "074800", "074820", "07413B", "074100", "07423B", "074200", "07433B", "074300"], index="CP Setting") -> (element=w170:string)
          n82 = call "WSVCAP SHL Host TL RFFE Write - Multiple DUTs - Common Data.vi"("Data Out"=w170, "error in"=w167, "Log (T)"=FALSE) -> ("error out"=w165:errorcluster)  [unwired: 12 in]
        }
      }
      n83 = Array Subset(array="Post CMd Delay", length="No of Cmd") -> (w105:dbl[])  [unwired: 1 in]
      n84 = Array Subset(array="Command", length="No of Cmd") -> (w106:string[])  [unwired: 1 in]
      n85 = property on="Post CMd Delay" class="Arr (strict)"("Number of Rows"="No of Cmd") -> ()  [unwired: 2 in, 2 out]
      n86 = local write "Command"(w106) -> ()
      n87 = local write "Post CMd Delay"(w105) -> ()
      n88 = property on="Command" class="Arr (strict)"("Number of Rows"="No of Cmd") -> ()  [unwired: 2 in, 2 out]
      n89 = Wait Until Next ms Multiple(millisecond multiple=u32 100) -> ()  [unwired: 1 out]
    }
    n90 = case shown="False" w80 {
      tunnel: w72 -> [w320 w1833]
      tunnel: [w305 w1833] -> w71
      tunnel: w87 -> [w321 _]
      tunnel: w74 -> [w319 w1831]
      tunnel: w73 -> [w311 w1832]
      tunnel: [w317 w1832] -> w85
      tunnel: [w315 w1831] -> w84
      tunnel: w82 -> [w308 w1830]
      tunnel: [w304 w1830] -> w81
      tunnel: "RFFE Slave Address" -> [w299 _]
      tunnel: [FALSE ("stop During HD/Cycles") FALSE ("stop During HD/Cycles")] -> w70
      tunnel: w69 -> [w274 _]
      tunnel: w68 -> [w273 _]
      tunnel: w67 -> [w272 _]
      tunnel: w66 -> [w271 _]
      tunnel: w65 -> [w270 _]
      tunnel: w64 -> [w269 _]
      tunnel: w63 -> [w268 _]
      tunnel: w61 -> [w262 _]
      tunnel: w60 -> [w261 _]
      frame False {
        w300 = u64 0 ("Total Completed")
        w279 = u32 100 ("milliseconds to wait")
        w316 = T7 [enum."Voltage 2", enum."Voltage 3", enum."Voltage 1"] items=["Idle...", "Voltage 1", "Voltage 2", "Voltage 3"]
        w318 = T7 [enum."Voltage 2", enum."Voltage 3", enum."Voltage 1"] items=["Idle...", "Voltage 1", "Voltage 2", "Voltage 3"]
        # "VSA"
        # "HS"
        # "HD/CYC"
        # "DVA"
        # "E-CAL"
        # "VPI"
        # "Verify Socket"
        n91 = for {
          tunnel: w320 -> [w1828]
          tunnel: w319 -> [w1827]
          tunnel: w318 -> [w1825] mode=indexing
          tunnel: [w1820] -> w313
          tunnel: [w1824] -> w303
          n92 = local read "Set VDD"() -> (w1823:dbl)
          n93 = call "E3631A_Voltage Controller updated.vi"("VISA resource name"=w1827, "I_VDD(A)"=0.5, "Channel Controller"=w1825, "Voltage 1"=w1823, "Voltage 2"=3.3, "error in (no error)"=w1828, "I_3.3V (A)"=0.5) -> ("VISA resource name out"=w1824:refnum<visa-resource-name>, "error out"=w1821:errorcluster)  [unwired: 7 in]
          n94 = call "Delay T4.vi"("milliseconds to wait"=u32 100, "error in (no error)"=w1821) -> ("error out"=w1820:errorcluster)  [unwired: 9 in]
        }
        n95 = local write "Total Time"(w300) -> ()
        n96 = local write "TTCompleted"(w300) -> ()
        n97 = call "WSVCAP SHL Host TL RFFE Write - Multiple DUTs - Common Data.vi"("Data Out"="074000", "error in"=w313, "Log (T)"=FALSE) -> ("error out"=w314:errorcluster)  [unwired: 12 in]
        n98 = local read "IDD Brd(uA)"() -> (w288:string)
        n99 = call "Delay T4.vi"("milliseconds to wait"=w279, "error in (no error)"=w314) -> ("error out"=w312:errorcluster)  [unwired: 9 in]
        n100 = call "Ke2000 Single Reading.vi"("error in (no error)"=w312, "VISA resource name"=w311) -> ("error out"=w289:errorcluster, "VISA resource name out"=w310:refnum<visa-resource-name>, "uA"=w291:string)  [unwired: 5 in, 2 out]
        n101 = call "Substration.vi"("error in (no error)"=w289, "Input2"=w288, "Input1"=w291) -> ("error out"=w264:errorcluster, "In1 - In2"=w290:string)  [unwired: 7 in]
        "IDD Stdby(uA)" <- w290
        n102 = case shown="True" w273 {
          tunnel: [1 ("X Repeat") w382] -> w302
          frame False {
          }
          frame True {
            n103 = local read "X Repeat"() -> (w382:i32)
          }
        }
        n104 = call "WSVCAP SHL Host TL RFFE Write - Multiple DUTs - Common Data.vi"("Data Out"="074040", "error in"=w264, "Log (T)"=FALSE) -> ("error out"=w263:errorcluster)  [unwired: 12 in]
        n105 = call "Delay T4.vi"("milliseconds to wait"=w279, "error in (no error)"=w263) -> ("error out"=w297:errorcluster)  [unwired: 9 in]
        n106 = case shown="False" w271 {
          tunnel: w297 -> [w344 w353]
          tunnel: [w343 w351] -> w295
          tunnel: ["DVA OFF" ("Data Out") "DVA ON" ("Data Out")] -> w296
          frame False {
            n107 = call "WSVCAP SHL Host TL RFFE Write - Multiple DUTs - Common Data.vi"("Data Out"="074820", "error in"=w344) -> ("error out"=w343:errorcluster)  [unwired: 13 in]
          }
          frame True {
            n108 = call "WSVCAP SHL Host TL RFFE Write - Multiple DUTs - Common Data.vi"("Data Out"="074800", "error in"=w353, "Log (T)"=FALSE) -> ("error out"=w349:errorcluster)  [unwired: 12 in]
            n109 = case shown="2" "CP with DVA ON" {
              selector: "CP with DVA ON" -> [w359 w364 w369 w374 w378]
              tunnel: string[] ["07442F", "074436", "074428", "074429", "07443B"] -> [w360 w365 w370 w375 w380]
              tunnel: [w358 w363 w368 w373 w379] -> w345
              tunnel: ["35.0" ("Data Out") "29.75" ("Data Out") "30.5" ("Data Out") "44.0" ("Data Out") "40.25" ("Data Out")] -> _
              tunnel: w349 -> [w356 w361 w366 w371 w376]
              tunnel: [w356 w361 w366 w371 w376] -> w348
              frame 0, Default {
                n110 = Index Array(array=w360, index=w359) -> (element=w358:string)
              }
              frame 2 {
                n111 = Index Array(array=w365, index=w364) -> (element=w363:string)
              }
              frame 3 {
                n112 = Index Array(array=w370, index=w369) -> (element=w368:string)
              }
              frame 4 {
                n113 = Index Array(array=w375, index=w374) -> (element=w373:string)
              }
              frame 1 {
                n114 = Index Array(array=w380, index=w378) -> (element=w379:string)
              }
            }
            n115 = call "WSVCAP SHL Host TL RFFE Write - Multiple DUTs - Common Data.vi"("Data Out"=w345, "error in"=w348, "Log (T)"=FALSE) -> ("error out"=w351:errorcluster)  [unwired: 12 in]
          }
        }
        n116 = for {
          N: 36 -> [_]
          tunnel: "Serial Number" -> [w326]
          tunnel: [w324] -> w276 mode=indexing
          i -> [w323]
          n117 = Increment(x=w323) -> (x+1=w322:i32)
          n118 = Index Array(array=w326, index (row)=w322, index (col)=1 ("disabled index (col)")) -> (element=w324:string)
        }
        n119 = Not(x=w268) -> (.not. x?=w275:bool)
        n120 = Number To Fractional String(number="Set VDD", precision (6)=i16 2) -> (F-format string=w293:string)  [unwired: 2 in]
        n121 = call "Delay T4.vi"("milliseconds to wait"=w279, "error in (no error)"=w295) -> ("error out"=w283:errorcluster)  [unwired: 9 in]
        n122 = case shown="True" w272 {
          tunnel: w283 -> [w330 w332]
          tunnel: [w327 w331] -> w282
          tunnel: ["CAL OFF" ("Data Out") "CAL ON" ("Data Out")] -> w284
          frame False {
            n123 = call "WSVCAP SHL Host TL RFFE Write - Multiple DUTs - Common Data.vi"("Data Out"="074044", "error in"=w330) -> ("error out"=w327:errorcluster)  [unwired: 13 in]
          }
          frame True {
            n124 = for {
              tunnel: string[] ["074900", "074920", "074900"] -> [w340] mode=indexing
              tunnel: w332 -> [w337]
              tunnel: [w336] -> w331
              n125 = call "WSVCAP SHL Host TL RFFE Write - Multiple DUTs - Common Data.vi"("Data Out"=w340, "error in"=w337, "Log (T)"=FALSE) -> ("error out"=w339:errorcluster)  [unwired: 12 in]
              n126 = call "Delay T4.vi"("milliseconds to wait"=u32 10, "error in (no error)"=w339) -> ("error out"=w336:errorcluster)  [unwired: 9 in]
            }
          }
        }
        n127 = for {
          N: w302 -> [_]
          tunnel: w321 -> [w420]
          tunnel: [w416] -> w317
          tunnel: w290 -> [w415]
          tunnel: w310 -> [w414]
          tunnel: "TMN DC\\CAP Data Log File Path" -> [w413]
          tunnel: w308 -> [w411]
          tunnel: [w410] -> w306
          tunnel: w303 -> [w385]
          shift-right: [w405] -> _
          shift-left: u64 0 -> [w407]
          tunnel: w273 -> [w404]
          tunnel: w299 -> [w399]
          tunnel: w299 -> [w398]
          tunnel: w296 -> [w397]
          tunnel: w293 -> [w396]
          tunnel: [w395] -> w287
          tunnel: w284 -> [w394]
          tunnel: w282 -> [w393]
          tunnel: w271 -> [w392]
          tunnel: w274 -> [w390]
          tunnel: w270 -> [w389]
          tunnel: w275 -> [w388]
          tunnel: w269 -> [w387]
          tunnel: w276 -> [w386]
          tunnel: [w385] -> w265
          tunnel: w262 -> [w384]
          tunnel: w261 -> [w383]
          i -> [w403]
          stop <- w391 stop-if-true
          n128 = while {
            tunnel: w420 -> [w434]
            tunnel: w413 -> [w664]
            tunnel: "Lot#" -> [w663]
            tunnel: "Wafer#" -> [w662]
            tunnel: w386 -> [w661]
            tunnel: "Test Program" -> [w660]
            tunnel: w386 -> [w659]
            tunnel: "Comment" -> [w658]
            tunnel: "Lot#" -> [w657]
            tunnel: "Wafer#" -> [w656]
            tunnel: w414 -> [w653]
            tunnel: [w655] -> w416
            tunnel: w415 -> [w652]
            tunnel: w411 -> [w649]
            tunnel: [w648] -> w410
            tunnel: [w557] -> w401
            tunnel: w403 -> [w594]
            tunnel: [w585] -> w405
            tunnel: w407 -> [w584]
            shift-right: [w583] -> _
            shift-left: u64 0 -> [w484]
            tunnel: [w582] -> w400
            tunnel: w404 -> [w581]
            tunnel: w399 -> [w556]
            tunnel: w398 -> [w554]
            tunnel: w397 -> [w502]
            tunnel: w396 -> [w500]
            tunnel: [w481] -> w395
            tunnel: w394 -> [w487]
            tunnel: w393 -> [w435]
            tunnel: w392 -> [w486]
            tunnel: w390 -> [w478]
            tunnel: w389 -> [w477]
            tunnel: w388 -> [w472]
            tunnel: w387 -> [w466]
            tunnel: w384 -> [w442]
            tunnel: w383 -> [w441]
            i -> [w439]
            stop <- w595 stop-if-true
            n129 = Array Size(array=w434) -> (size(s)=w433:i32[])
            n130 = Index Array(array=w434, index (row)=w439, index (col)=0 ("disabled index (col)")) -> (element=w431:dbl)
            n131 = Index Array(array=w433, index=0) -> (element=w422:i32)
            n132 = call "CP_Cmd_Setting.vi"("error in (no error)"=w435, "Input"=w431) -> ("error out"=w438:errorcluster, "CP Voltage"=w436:string, "Send Cmd"=w437:string)  [unwired: 6 in, 1 out]
            "CP Voltage" <- w436
            n133 = To Unsigned Quad Integer(1:w422) -> (0:w421:u64)
            n134 = flat-sequence {
              tunnel: [w729] -> w647
              tunnel: [w726] -> w646
              tunnel: [w728] -> w645
              tunnel: w653 -> [w708]
              tunnel: w652 -> [w727]
              tunnel: [w727] -> w644
              tunnel: [w681] -> w643
              tunnel: [w678] -> w642
              tunnel: w438 -> [w721]
              tunnel: w594 -> [w724]
              tunnel: w439 -> [w704]
              tunnel: [w704] -> w591
              tunnel: w581 -> [w723]
              tunnel: [w722] -> w580
              tunnel: [w687] -> w575
              tunnel: [w686] -> w574
              tunnel: [w685] -> w573
              tunnel: [w691] -> w563
              tunnel: [w688] -> w562
              tunnel: w556 -> [w720]
              tunnel: [w720] -> w555
              tunnel: w554 -> [w719]
              tunnel: [w690] -> w541
              tunnel: [w689] -> w515
              tunnel: [w718] -> w503
              tunnel: w437 -> [w716]
              tunnel: [w705] -> w499
              tunnel: [w668] -> w491
              tunnel: w478 -> [w701]
              tunnel: w477 -> [w700]
              tunnel: [w700] -> w476
              tunnel: w472 -> [w699]
              tunnel: [w699] -> w471
              tunnel: w466 -> [w698]
              tunnel: [w698] -> w465
              tunnel: [w694] -> w460
              tunnel: ["Test Sequences"] -> w456
              tunnel: "Real No. From\nLookup Table" -> [w684]
              tunnel: ["WS1050/51"] -> w450
              tunnel: ["Cmin/Act"] -> w446
              tunnel: w442 -> [w673]
              tunnel: w441 -> [w672]
              tunnel: w431 -> [w671]
              tunnel: w421 -> [w665]
              tunnel: w431 -> [w666]
              tunnel: [w665] -> w430
              tunnel: w647 -> [w1020]
              tunnel: [w1016] -> w553
              tunnel: w646 -> [w1019]
              tunnel: w645 -> [w1025]
              tunnel: [w1025] -> w552
              tunnel: w644 -> [w1024]
              tunnel: w643 -> [w1018]
              tunnel: w642 -> [w1017]
              tunnel: [w1007] -> w551
              tunnel: [w1024] -> w550
              tunnel: [w1018] -> w549
              tunnel: [w1017] -> w548
              tunnel: w591 -> [w1022]
              tunnel: [w1022] -> w547
              tunnel: w580 -> [w1021]
              tunnel: [w1021] -> w546
              tunnel: [w1019] -> w545
              tunnel: w575 -> [w1015]
              tunnel: w574 -> [w1000]
              tunnel: w573 -> [w1001]
              tunnel: [w1012] -> w544
              tunnel: w563 -> [w1014]
              tunnel: w562 -> [w1012]
              tunnel: [w1008] -> w543
              tunnel: w555 -> [w1013]
              tunnel: [w998] -> w542
              tunnel: w541 -> [w998]
              tunnel: [w1000] -> w540
              tunnel: w515 -> [w999]
              tunnel: [w999] -> w514
              tunnel: [w1001] -> w512
              tunnel: w503 -> [w1011]
              tunnel: [w1010] -> w492
              tunnel: w491 -> [w1010]
              tunnel: w476 -> [w1006]
              tunnel: [w1006] -> w475
              tunnel: w471 -> [w1005]
              tunnel: [w1005] -> w470
              tunnel: w465 -> [w1004]
              tunnel: [w1004] -> w464
              tunnel: w460 -> [w1003]
              tunnel: [w1002] -> w459
              tunnel: w456 -> [w996]
              tunnel: [w996] -> w455
              tunnel: w450 -> [w995]
              tunnel: [w995] -> w449
              tunnel: w446 -> [w994]
              tunnel: [w994] -> w445
              tunnel: w430 -> [w993]
              tunnel: [w993] -> w429
              tunnel: w553 -> [w1140]
              tunnel: [w1139] -> w539
              tunnel: w552 -> [w1151]
              tunnel: [w1151] -> w536
              tunnel: w551 -> [w1131]
              tunnel: [w1131] -> w534
              tunnel: w550 -> [w1150]
              tunnel: [w1150] -> w532
              tunnel: w549 -> [w1149]
              tunnel: [w1149] -> w530
              tunnel: w548 -> [w1148]
              tunnel: [w1148] -> w528
              tunnel: w547 -> [w1147]
              tunnel: [w1147] -> w526
              tunnel: w546 -> [w1146]
              tunnel: [w1146] -> w524
              tunnel: w545 -> [w1145]
              tunnel: [w1145] -> w522
              tunnel: w544 -> [w1144]
              tunnel: [w1144] -> w520
              tunnel: [w1136] -> w518
              tunnel: w543 -> [w1135]
              tunnel: w542 -> [w1142]
              tunnel: w540 -> [w1141]
              tunnel: w514 -> [w1128]
              tunnel: [w1128] -> w513
              tunnel: w512 -> [w1130]
              tunnel: [w1130] -> w511
              tunnel: [w1137] -> w510
              tunnel: [w1138] -> w493
              tunnel: w492 -> [w1138]
              tunnel: w475 -> [w1134]
              tunnel: [w1134] -> w474
              tunnel: w470 -> [w1133]
              tunnel: [w1133] -> w469
              tunnel: w464 -> [w1132]
              tunnel: [w1132] -> w463
              tunnel: w459 -> [w1129]
              tunnel: w455 -> [w1126]
              tunnel: [w1129] -> w454
              tunnel: [w1126] -> w453
              tunnel: w449 -> [w1125]
              tunnel: [w1125] -> w448
              tunnel: w445 -> [w1124]
              tunnel: [w1124] -> w444
              tunnel: w429 -> [w1123]
              tunnel: [w1123] -> w428
              tunnel: w539 -> [w1233]
              tunnel: [w1232] -> w538
              tunnel: [w1228] -> w537
              tunnel: w536 -> [w1245]
              tunnel: [w1245] -> w535
              tunnel: w534 -> [w1222]
              tunnel: [w1222] -> w533
              tunnel: w532 -> [w1244]
              tunnel: [w1244] -> w531
              tunnel: w530 -> [w1243]
              tunnel: [w1243] -> w529
              tunnel: w528 -> [w1242]
              tunnel: [w1242] -> w527
              tunnel: w526 -> [w1241]
              tunnel: [w1241] -> w525
              tunnel: w524 -> [w1240]
              tunnel: [w1240] -> w523
              tunnel: w522 -> [w1239]
              tunnel: [w1239] -> w521
              tunnel: w520 -> [w1238]
              tunnel: [w1238] -> w519
              tunnel: w518 -> [w1237]
              tunnel: [w1237] -> w517
              tunnel: [w1219] -> w516
              tunnel: w513 -> [w1235]
              tunnel: w511 -> [w1234]
              tunnel: w510 -> [w1227]
              tunnel: ["DeltaC Target Setting(pF)"] -> w501
              tunnel: [w1230] -> w494
              tunnel: w493 -> [w1230]
              tunnel: w486 -> [w1229]
              tunnel: [w1229] -> w485
              tunnel: w474 -> [w1226]
              tunnel: [w1226] -> w473
              tunnel: w469 -> [w1225]
              tunnel: [w1225] -> w468
              tunnel: w463 -> [w1224]
              tunnel: [w1224] -> w462
              tunnel: w454 -> [w1223]
              tunnel: w453 -> [w1220]
              tunnel: [w1219] -> w451
              tunnel: w448 -> [w1218]
              tunnel: [w1218] -> w447
              tunnel: w444 -> [w1217]
              tunnel: [w1217] -> w443
              tunnel: w428 -> [w1216]
              tunnel: [w1216] -> w427
              tunnel: [w1364] -> w641
              tunnel: [w1330] -> w640
              tunnel: w538 -> [w1368]
              tunnel: w537 -> [w1344]
              tunnel: [w1353] -> w639
              tunnel: [w1344] -> w638
              tunnel: [w1367] -> w637
              tunnel: [w1366] -> w636
              tunnel: w535 -> [w1365]
              tunnel: [w1365] -> w635
              tunnel: w533 -> [w1353]
              tunnel: w531 -> [w1363]
              tunnel: [w1363] -> w634
              tunnel: w529 -> [w1359]
              tunnel: [w1359] -> w633
              tunnel: w527 -> [w1358]
              tunnel: [w1358] -> w632
              tunnel: w525 -> [w1354]
              tunnel: [w1354] -> w590
              tunnel: w523 -> [w1362]
              tunnel: [w1362] -> w579
              tunnel: w521 -> [w1361]
              tunnel: [w1360] -> w576
              tunnel: w519 -> [w1356]
              tunnel: w517 -> [w1352]
              tunnel: [w1357] -> w572
              tunnel: [w1355] -> w571
              tunnel: [w1352] -> w566
              tunnel: w516 -> [w1351]
              tunnel: [w1338] -> w561
              tunnel: [w1337] -> w560
              tunnel: [w1336] -> w559
              tunnel: w501 -> [w1350]
              tunnel: [w1335] -> w495
              tunnel: w494 -> [w1335]
              tunnel: [w1334] -> w490
              tunnel: w485 -> [w1333]
              tunnel: w473 -> [w1328]
              tunnel: w468 -> [w1327]
              tunnel: [w1327] -> w467
              tunnel: w462 -> [w1326]
              tunnel: [w1326] -> w461
              tunnel: w451 -> [w1323]
              tunnel: w447 -> [w1322]
              tunnel: w443 -> [w1311]
              tunnel: w427 -> [w1310]
              tunnel: [w1310] -> w426
              tunnel: w641 -> [w1572]
              tunnel: [w1572] -> w631
              tunnel: [w1557] -> w630
              tunnel: [w1571] -> w629
              tunnel: w640 -> [w1570]
              tunnel: w639 -> [w1569]
              tunnel: w638 -> [w1568]
              tunnel: [w1569] -> w628
              tunnel: [w1568] -> w627
              tunnel: w637 -> [w1567]
              tunnel: [w1567] -> w626
              tunnel: w636 -> [w1566]
              tunnel: [w1566] -> w625
              tunnel: w635 -> [w1565]
              tunnel: [w1565] -> w624
              tunnel: w634 -> [w1564]
              tunnel: [w1564] -> w623
              tunnel: w633 -> [w1563]
              tunnel: [w1563] -> w622
              tunnel: w632 -> [w1562]
              tunnel: [w1562] -> w621
              tunnel: w649 -> [w1561]
              tunnel: [w1559] -> w620
              tunnel: [w1539] -> w619
              tunnel: [w1540] -> w618
              tunnel: [w1538] -> w617
              tunnel: w590 -> [w1555]
              tunnel: [w1555] -> w589
              tunnel: w579 -> [w1554]
              tunnel: [w1554] -> w578
              tunnel: w576 -> [w1571]
              tunnel: w572 -> [w1552]
              tunnel: w571 -> [w1553]
              tunnel: [w1553] -> w570
              tunnel: [w1552] -> w568
              tunnel: w566 -> [w1551]
              tunnel: [w1551] -> w565
              tunnel: w561 -> [w1537]
              tunnel: w560 -> [w1536]
              tunnel: w559 -> [w1535]
              tunnel: [w1532] -> w558
              tunnel: [w1537] -> w509
              tunnel: [w1536] -> w507
              tunnel: [w1535] -> w505
              tunnel: [w1534] -> w496
              tunnel: w495 -> [w1534]
              tunnel: w490 -> [w1533]
              tunnel: [w1533] -> w489
              tunnel: w467 -> [w1532]
              tunnel: w461 -> [w1531]
              tunnel: w426 -> [w1530]
              tunnel: [w1530] -> w425
              tunnel: w631 -> [w1668]
              tunnel: [w1668] -> w616
              tunnel: w630 -> [w1692]
              tunnel: [w1691] -> w615
              tunnel: w664 -> [w1693]
              tunnel: w663 -> [w1690]
              tunnel: w662 -> [w1689]
              tunnel: w661 -> [w1688]
              tunnel: [w1687] -> w614
              tunnel: w629 -> [w1681]
              tunnel: [w1681] -> w613
              tunnel: w628 -> [w1686]
              tunnel: w627 -> [w1685]
              tunnel: [w1686] -> w612
              tunnel: [w1685] -> w611
              tunnel: [w1676] -> w610
              tunnel: w626 -> [w1684]
              tunnel: [w1684] -> w609
              tunnel: w625 -> [w1683]
              tunnel: [w1683] -> w608
              tunnel: w624 -> [w1680]
              tunnel: [w1682] -> w607
              tunnel: w484 -> [w1679]
              tunnel: [w1678] -> w606
              tunnel: [w1666] -> w605
              tunnel: w623 -> [w1677]
              tunnel: w622 -> [w1675]
              tunnel: w621 -> [w1674]
              tunnel: "File Name" -> [w1673]
              tunnel: w620 -> [w1672]
              tunnel: [w1672] -> w604
              tunnel: w619 -> [w1671]
              tunnel: [w1671] -> w603
              tunnel: [w1670] -> w602
              tunnel: w618 -> [w1670]
              tunnel: w617 -> [w1669]
              tunnel: [w1669] -> w601
              tunnel: [w1664] -> w592
              tunnel: w589 -> [w1665]
              tunnel: [w1665] -> w587
              tunnel: w584 -> [w1663]
              tunnel: w578 -> [w1662]
              tunnel: [w1662] -> w577
              tunnel: w570 -> [w1661]
              tunnel: [w1661] -> w569
              tunnel: w568 -> [w1660]
              tunnel: [w1660] -> w567
              tunnel: w565 -> [w1659]
              tunnel: [w1659] -> w564
              tunnel: w558 -> [w1658]
              tunnel: w509 -> [w1657]
              tunnel: [w1657] -> w508
              tunnel: w507 -> [w1656]
              tunnel: [w1656] -> w506
              tunnel: w505 -> [w1655]
              tunnel: [w1655] -> w504
              tunnel: w499 -> [w1654]
              tunnel: [w1654] -> w498
              tunnel: [w1653] -> w497
              tunnel: w496 -> [w1653]
              tunnel: w489 -> [w1652]
              tunnel: [w1652] -> w488
              tunnel: ["Freq(Hz)"] -> w458
              tunnel: ["Board#"] -> w457
              tunnel: w425 -> [w1649]
              tunnel: [w1649] -> w424
              tunnel: w616 -> [w1766]
              tunnel: w615 -> [w1765]
              tunnel: w664 -> [w1728]
              tunnel: w660 -> [w1760]
              tunnel: w659 -> [w1763]
              tunnel: w658 -> [w1759]
              tunnel: w657 -> [w1762]
              tunnel: w656 -> [w1758]
              tunnel: w614 -> [w1761]
              tunnel: [w1766] -> w597
              tunnel: [w1764] -> w598
              tunnel: w613 -> [w1756]
              tunnel: [w1756] -> w599
              tunnel: w612 -> [w1755]
              tunnel: w611 -> [w1740]
              tunnel: w610 -> [w1754]
              tunnel: w609 -> [w1753]
              tunnel: w608 -> [w1742]
              tunnel: [w1750] -> w600
              tunnel: w607 -> [w1752]
              tunnel: w606 -> [w1751]
              tunnel: w605 -> [w1750]
              tunnel: "File Name" -> [w1721]
              tunnel: w604 -> [w1749]
              tunnel: [w1749] -> w596
              tunnel: w603 -> [w1748]
              tunnel: w602 -> [w1747]
              tunnel: w601 -> [w1746]
              tunnel: [w1745] -> w593
              tunnel: w592 -> [w1745]
              tunnel: [w1724] -> w588
              tunnel: w587 -> [w1724]
              tunnel: w577 -> [w1744]
              tunnel: w569 -> [w1743]
              tunnel: w567 -> [w1741]
              tunnel: w564 -> [w1739]
              tunnel: w508 -> [w1738]
              tunnel: w506 -> [w1737]
              tunnel: w504 -> [w1736]
              tunnel: w502 -> [w1735]
              tunnel: w487 -> [w1734]
              tunnel: w436 -> [w1733]
              tunnel: w500 -> [w1732]
              tunnel: w498 -> [w1731]
              tunnel: w497 -> [w1730]
              tunnel: w488 -> [w1729]
              tunnel: [w1726] -> w483
              tunnel: [w1717] -> w479
              tunnel: w458 -> [w1716]
              tunnel: w457 -> [w1714]
              tunnel: w424 -> [w1713]
              tunnel: [w1713] -> w423
              tunnel: [w1787] -> w654
              tunnel: [w1788] -> w655
              tunnel: [w1789] -> w557
              tunnel: w600 -> [w1780]
              tunnel: w599 -> [w1788]
              tunnel: w598 -> [w1777]
              tunnel: w597 -> [w1789]
              tunnel: w596 -> [w1782]
              tunnel: [w1782] -> w648
              tunnel: [w1779] -> w585
              tunnel: w593 -> [w1779]
              tunnel: w588 -> [w1781]
              tunnel: [w1781] -> w586
              tunnel: [w1780] -> w583
              tunnel: [w1778] -> w582
              tunnel: [w1776] -> w480
              tunnel: w483 -> [w1775]
              tunnel: w479 -> [w1773]
              tunnel: w423 -> [w1772]
              frame #0 {
                w695 = FALSE ("Log (T)")
                n135 = call "WSVCAP SHL Host TL RFFE Write - Multiple DUTs - Common Data.vi"("Data Out"=w716, "error in"=w721, "Log (T)"=FALSE) -> ("error out"=w702:errorcluster)  [unwired: 12 in]
                n136 = for {
                  tunnel: string[] ["0760", "0767", "0768"] -> [w751] mode=indexing
                  tunnel: [w747] -> w706 mode=indexing
                  tunnel: w702 -> [w745]
                  tunnel: [w744] -> w703
                  i -> [w750]
                  n137 = call "Delay T4.vi"("milliseconds to wait"=u32 10, "error in (no error)"=w745) -> ("error out"=w752:errorcluster)  [unwired: 9 in]
                  n138 = call "WSVCAP SHL Host TL RFFE Read - Multiple DUTs - Common Data.vi"("Data Out"=w751, "error in"=w752, "Log (T)"=FALSE) -> ("RFFE Data In"=w749:string[], "error out"=w744:errorcluster)  [unwired: 11 in]
                  n139 = Index Array(array=w749, index=w750) -> (element=w746:string)
                  n140 = String Subset(string=w746, offset (0)=0) -> (substring=w747:string)  [unwired: 1 in]
                }
                "RB Reg for HD/Cycle" <- w706
                n141 = local read "IDD Brd(uA)"() -> (w715:string)
                n142 = call "Delay T4.vi"("milliseconds to wait"=u32 100, "error in (no error)"=w703) -> ("error out"=w711:errorcluster)  [unwired: 9 in]
                n143 = call "Ke2000 Single Reading.vi"("error in (no error)"=w711, "VISA resource name"=w708) -> ("error out"=w713:errorcluster, "VISA resource name out"=w683:refnum<visa-resource-name>, "uA"=w714:string)  [unwired: 5 in, 2 out]
                n144 = call "Substration.vi"("error in (no error)"=w713, "Input2"=w715, "Input1"=w714) -> ("error out"=w710:errorcluster, "In1 - In2"=→"IDD_HD/CYC (uA)":string)  [unwired: 7 in]
                n145 = case shown="False" w723 {
                  tunnel: [w783 w888] -> w729
                  tunnel: [w784 w873] -> w667
                  tunnel: [w782 w889] -> w728
                  tunnel: w710 -> [w778 w877]
                  tunnel: w724 -> [_ w879]
                  tunnel: w671 -> [w775 w874]
                  tunnel: [w780 w875] -> w722
                  tunnel: w704 -> [w767 w871]
                  tunnel: w719 -> [w777 _]
                  tunnel: ["% Duty Cycle" "100" ("Data Out")] -> w705
                  tunnel: w701 -> [w765 _]
                  tunnel: w684 -> [w764 w866]
                  tunnel: w673 -> [w761 _]
                  tunnel: w672 -> [w760 _]
                  frame False {
                    # "Cycles in 1s"
                    n146 = case shown="True" w764 {
                      tunnel: w778 -> [w790 w796]
                      tunnel: w775 -> [w789 w795]
                      tunnel: [w788 w796] -> w774
                      tunnel: w767 -> [w787 _]
                      tunnel: [w786 w795] -> w773
                      tunnel: [u64 1000 ("y") u64 1 ("y")] -> w768
                      frame False {
                        n147 = case shown="8, Default" w787 {
                          tunnel: w789 -> [w792 _]
                          tunnel: [w792 "Cycle RP"] -> w786
                          tunnel: [w791 w793] -> w788
                          tunnel: w790 -> [w791 w793]
                          frame 0..7 {
                          }
                          frame 8, Default {
                          }
                        }
                      }
                      frame True {
                        # "Read real number\nfrom lookup table"
                      }
                    }
                    n148 = call "WSVCAP SHL Host TL RFFE Configure.vi"("RFFE Slave Address"=w777, "Clock Rate (Hz)"="SPI Clock Rate (Hz)", "error in"=w774) -> ("Actual Rate (Hz)"=→"AR Cycling(Hz)":dbl, "error out"=w763:errorcluster)  [unwired: 11 in]
                    n149 = Array Max & Min(array=w760) -> (max value=w771:dbl)  [unwired: 3 out]
                    n150 = Divide(x=1.0, y=w771) -> (x/y=w770:dbl)
                    n151 = To Unsigned Quad Integer(1:w770) -> (0:w769:u64)
                    n152 = Not(x=w765) -> (.not. x?=w766:bool)
                    n153 = case shown="False" w766 {
                      tunnel: [w799 w821] -> w784
                      tunnel: [w802 w820] -> w783
                      tunnel: [u64 1 w819] -> w782
                      tunnel: w763 -> [w800 w818]
                      tunnel: w773 -> [_ w817]
                      tunnel: w760 -> [_ w815]
                      tunnel: w769 -> [_ w814]
                      tunnel: w768 -> [_ w813]
                      tunnel: w767 -> [w798 _]
                      tunnel: w761 -> [_ w812]
                      frame False {
                        n154 = case shown="1, Default" w798 {
                          tunnel: w800 -> [w803 w805]
                          tunnel: [w803 w804] -> w799
                          frame 0 {
                          }
                          frame 1, Default {
                            n155 = flat-sequence {
                              tunnel: "Repeat Meas(s)" -> [w811]
                              tunnel: w805 -> [w808]
                              tunnel: [w808] -> w804
                              frame #0 {
                                n156 = Multiply(x=w811, y=u32 1000) -> (x*y=w810:u32)
                                n157 = Wait (ms)(milliseconds to wait=w810) -> ()  [unwired: 1 out]
                                n158 = local write "STATUS"("Verify Sockets waiting times..." ("STATUS")) -> ()
                              }
                            }
                          }
                        }
                        n159 = local read "stop During HD/Cycles"() -> (w802:bool)
                      }
                      frame True {
                        n160 = while {
                          tunnel: w817 -> [w841]
                          tunnel: [w828] -> w821
                          tunnel: [w833] -> w820
                          tunnel: w818 -> [w839]
                          tunnel: [w827] -> w819
                          tunnel: w812 -> [w838]
                          tunnel: w815 -> [w837]
                          tunnel: w814 -> [w824]
                          tunnel: w813 -> [w822]
                          i -> [w836]
                          stop <- w832 stop-if-true
                          # "At least 1 second before target"
                          # "Remaining Cycles"
                          # "Target Cycles"
                          # "Cycles in 1s"
                          n161 = To Unsigned Quad Integer(1:w841) -> (0:w840:u64)
                          n162 = case shown="0" w836 {
                            tunnel: [w849 w851] -> w830
                            tunnel: w839 -> [w850 w851]
                            tunnel: w838 -> [w848 _]
                            tunnel: w837 -> [w847 _]
                            frame 0 {
                              n163 = call "WSVCAP SHL Host TL RFFE Write Cycle - Multiple DUTs - Common Data.vi"("Data Out (Cycle Commands)"=w848, "Post Command Delay"=w847, "error in"=w850, "Log (T)"=FALSE) -> ("error out"=w849:errorcluster)  [unwired: 11 in]
                            }
                            frame 1, Default {
                            }
                          }
                          n164 = Multiply(x=w840, y=w822) -> (x*y=w827:u64)
                          n165 = call "WSVCAP SHL Host TL SPI_RFFE Query Cycle Count.vi"("error in"=w830) -> ("Cycle Count"=w826:u64, "error out"=w835:errorcluster)  [unwired: 13 in]
                          "Cycle Count" <- w826
                          n166 = Subtract(x=w827, y=w826) -> (x-y=w825:u64)
                          n167 = Greater Or Equal?(x=w826, y=w827) -> (x >= y?=w834:bool)
                          n168 = local read "stop During HD/Cycles"() -> (w833:bool)
                          n169 = Greater?(x=w825, y=w824) -> (0:w823:bool)
                          n170 = case shown="True" w834 {
                            tunnel: [w853 w856] -> w829
                            tunnel: w835 -> [w853 w855]
                            tunnel: [FALSE TRUE] -> w831
                            frame False {
                            }
                            frame True {
                              n171 = call "WSVCAP SHL Host TL SPI Stop Write Cycle.vi"("error in"=w855) -> ("error out"=w856:errorcluster)  [unwired: 14 in]
                            }
                          }
                          n172 = Or(x=w831, y=w833) -> (x .or. y?=w832:bool)
                          n173 = case shown="True" w823 {
                            tunnel: w829 -> [w842 w845]
                            tunnel: [w842 w844] -> w828
                            frame False {
                            }
                            frame True {
                              n174 = call "MISC Wait with Data Flow.vi"("Error In (no error)"=w845, "Wait Time (500ms)"=u32 50) -> ("Error Out"=w844:errorcluster)  [unwired: 7 in, 2 out]
                            }
                          }
                        }
                        n175 = local write "STATUS"("Parts are Cycling...." ("STATUS")) -> ()
                      }
                    }
                    n176 = local read "HD/CYC Temp"() -> (w779:i32)
                    n177 = Number To Engineering String(4:w779) -> (0:w780:string)  [unwired: 3 in]
                  }
                  frame True {
                    n178 = case shown="False" w866 {
                      tunnel: w879 -> [w906 _]
                      tunnel: [w905 w918] -> w878
                      tunnel: w877 -> [w904 w919]
                      tunnel: [w903 w919] -> w876
                      tunnel: w874 -> [w902 w918]
                      tunnel: w871 -> [w901 _]
                      frame False {
                        n179 = case shown="1, Default" w906 {
                          tunnel: [w909 w916] -> w905
                          tunnel: w904 -> [w911 w917]
                          tunnel: [w910 w917] -> w903
                          tunnel: w902 -> [w908 _]
                          tunnel: w901 -> [w907 _]
                          frame 0 {
                            n180 = case shown="15, Default" w907 {
                              tunnel: [w912 "HD RP"] -> w909
                              tunnel: w911 -> [w913 w914]
                              tunnel: [w913 w914] -> w910
                              tunnel: w908 -> [w912 _]
                              frame 0..14 {
                              }
                              frame 15, Default {
                              }
                            }
                          }
                          frame 1, Default {
                            n181 = local read "HD RP"() -> (w916:dbl)
                          }
                        }
                      }
                      frame True {
                      }
                    }
                    n182 = call "WSVCAP SHL Host TL RFFE Write - Multiple DUTs - Common Data.vi"("Data Out"="Cmd To HD", "error in"=w876, "Log (T)"=FALSE) -> ("error out"=w862:errorcluster)  [unwired: 12 in]
                    n183 = local read "No of HD/Cycle\nCompleted"() -> (w880:u64)
                    n184 = call "Delay T4.vi"("milliseconds to wait"=u32 50, "error in (no error)"=w862) -> ("error out"=w859:errorcluster)  [unwired: 9 in]
                    n185 = for {
                      tunnel: string[] ["0761", "0762", "0763"] -> [w900] mode=indexing
                      tunnel: [w896] -> w858 mode=indexing
                      shift-right: [w893] -> w884
                      shift-left: w859 -> [w899]
                      i -> [w898]
                      n186 = call "WSVCAP SHL Host TL RFFE Read - Multiple DUTs - Common Data.vi"("Data Out"=w900, "error in"=w899, "Log (T)"=FALSE) -> ("RFFE Data In"=w895:string[], "error out"=w892:errorcluster)  [unwired: 11 in]
                      n187 = Index Array(array=w895, index=w898) -> (element=w894:string)
                      n188 = call "Delay T4.vi"("milliseconds to wait"=u32 10, "error in (no error)"=w892) -> ("error out"=w893:errorcluster)  [unwired: 9 in]
                      n189 = String Subset(string=w894, offset (0)=0) -> (substring=w896:string)  [unwired: 1 in]
                    }
                    "RB Reg for HD" <- w858
                    n190 = Greater?(x="HD_DC (Min)", y=w880) -> (0:w881:bool)
                    n191 = case shown="True" w881 {
                      tunnel: [_ w930] -> w886
                      tunnel: [w921 w929] -> w885
                      tunnel: w884 -> [w921 w928]
                      tunnel: w878 -> [w920 w927]
                      tunnel: [w920 w927] -> w883
                      frame False {
                      }
                      frame True {
                        n192 = Multiply(x=1000.0, y=w927) -> (x*y=w925:dbl)
                        n193 = Multiply(x=60.0, y=w925) -> (x*y=w923:dbl)
                        n194 = local write "STATUS"("Parts are Holding Down..." ("STATUS")) -> ()
                        n195 = event shown="[0] Timeout" {
                          selector: _ -> [_ _]
                          dyn-events: _ -> [_ _]
                          timeout: w923 -> [_ _]
                          tunnel: ["stop During HD/Cycles" TRUE ("stop During HD/Cycles")] -> w930
                          tunnel: w928 -> [w931 w933]
                          tunnel: [w931 w933] -> w929
                          event Timeout {
                            n196 = event-data() -> ()  [unwired: 1 in, 2 out]
                          }
                          event "stop During HD/Cycles": Value Change {
                            n197 = event-data() -> ()  [unwired: 1 in, 2 out]
                          }
                        }
                      }
                    }
                    n198 = Greater Or Equal?(x=w880, y="HD_DC (Min)") -> (x >= y?=w887:bool)
                    n199 = To Unsigned Quad Integer(1:w878) -> (0:w889:u64)
                    n200 = Add(x="Time All OFF (s)", y="Time All ON (s)") -> (x+y=w868:u32)
                    n201 = To Double Precision Float(number=w868) -> (double precision float=w867:dbl)
                    n202 = Divide(x=w867, y=60.0) -> (x/y=w869:dbl)
                    n203 = case shown="False" w887 {
                      tunnel: [w937 w953] -> w888
                      tunnel: [w938 w945] -> w873
                      tunnel: w885 -> [w938 w952]
                      tunnel: w886 -> [w937 w951]
                      tunnel: w883 -> [_ w950]
                      tunnel: [w936 w948] -> w875
                      tunnel: w869 -> [_ w942]
                      tunnel: "Time All OFF (s)" -> [_ w940]
                      tunnel: "Time All ON (s)" -> [_ w939]
                      frame False {
                        n204 = Number To Engineering String(4:"HD/CYC Temp") -> (0:w936:string)  [unwired: 3 in]
                      }
                      frame True {
                        n205 = Divide(x=w950, y=w942) -> (x/y=w949:dbl)
                        n206 = call "WSVCAP SHL Host TL RFFE Write - Multiple DUTs - Common Data.vi"("Data Out"="070201000000", "error in"=w952, "Log (T)"=FALSE) -> ("error out"=w955:errorcluster)  [unwired: 12 in]
                        n207 = Round To Nearest(number=w949) -> (nearest integer value=w944:dbl)
                        n208 = call "Delay T4.vi"("milliseconds to wait"=u32 50, "error in (no error)"=w955) -> ("error out"=w946:errorcluster)  [unwired: 9 in]
                        n209 = To Long Integer(number=w944) -> (32bit integer=w943:i32)
                        "No LPs to RP" <- w943
                        n210 = for {
                          N: w943 -> [_]
                          tunnel: w951 -> [w973]
                          tunnel: [w972] -> w953
                          tunnel: w946 -> [w962]
                          tunnel: [w961] -> w945
                          tunnel: w940 -> [w959]
                          tunnel: w939 -> [w957]
                          i -> [w971]
                          stop <- w972 stop-if-true
                          w960 = FALSE ("Log (T)")
                          w958 = u32 1 ("milliseconds to wait")
                          n211 = Increment(x=w971) -> (x+1=→"LPs Count":i32)
                          n212 = call "WSVCAP SHL Host TL RFFE Write - Multiple DUTs - Common Data.vi"("Data Out"="074776", "error in"=w962, "Log (T)"=w960) -> ("error out"=w979:errorcluster)  [unwired: 12 in]
                          n213 = call "Delay T4.vi"("milliseconds to wait"=w958, "error in (no error)"=w979) -> ("error out"=w978:errorcluster)  [unwired: 9 in]
                          n214 = local read "Set CP to Meas"() -> (w964:i32)
                          n215 = call "WSVCAP SHL Host TL RFFE Write - Multiple DUTs - Common Data.vi"("Data Out"="070201000000", "error in"=w965) -> ("error out"=w975:errorcluster)  [unwired: 13 in]
                          n216 = call "WSVCAP SHL Host TL RFFE Write - Multiple DUTs - Common Data.vi"("Data Out"="0702013B3B3B", "error in"=w978, "Log (T)"=w960) -> ("error out"=w968:errorcluster)  [unwired: 12 in]
                          n217 = call "Delay T4.vi"("milliseconds to wait"=w958, "error in (no error)"=w968) -> ("error out"=w967:errorcluster)  [unwired: 9 in]
                          n218 = flat-sequence {
                            tunnel: w975 -> [w986]
                            tunnel: [w984] -> w961
                            tunnel: w959 -> [w981]
                            frame #0 {
                              n219 = local write "STATUS"("Now HD OFF Time..." ("STATUS")) -> ()
                              n220 = Multiply(x=w981, y=u32 1000) -> (x*y=w983:u32)
                              n221 = call "Delay T4.vi"("milliseconds to wait"=w983, "error in (no error)"=w986) -> ("error out"=w984:errorcluster)  [unwired: 9 in]
                            }
                          }
                          n222 = Index Array(array=string[] ["07476F", "074776", "074765", "074769", "07477B"], index=w964) -> (element=w969:string)
                          n223 = call "WSVCAP SHL Host TL RFFE Write - Multiple DUTs - Common Data.vi"("Data Out"=w969, "error in"=w967, "Log (T)"=w960) -> ("error out"=w966:errorcluster)  [unwired: 12 in]
                          n224 = flat-sequence {
                            tunnel: [w991] -> w965
                            tunnel: w966 -> [w988]
                            tunnel: w957 -> [w987]
                            frame #0 {
                              n225 = local write "STATUS"("Now HD ON Time..." ("STATUS")) -> ()
                              n226 = Multiply(x=w987, y=u32 1000) -> (x*y=w990:u32)
                              n227 = call "Delay T4.vi"("milliseconds to wait"=w990, "error in (no error)"=w988) -> ("error out"=w991:errorcluster)  [unwired: 9 in]
                            }
                          }
                          n228 = Unbundle By Name(w961) -> ("status"=w974:bool)
                          n229 = Or(x=w974, y=w973) -> (x .or. y?=w972:bool)
                        }
                        n230 = Number To Engineering String(4:"DC_Temp") -> (0:w948:string)  [unwired: 3 in]
                      }
                    }
                  }
                }
                n231 = call "CP_Cmd_Setting.vi"("error in (no error)"=w667, "Input"=w666) -> ("error out"=w670:errorcluster, "CP Voltage"=w668:string, "Send Cmd"=w669:string)  [unwired: 6 in, 1 out]
                n232 = flat-sequence {
                  tunnel: w697 -> [w754]
                  tunnel: [w754] -> w693
                  frame #0 {
                    w756 = "0" ("NOM IDD OFF(uA)")
                    w757 = string[] []
                    w758 = string[][] []
                    n233 = local write "Total Delta C1(pF)"(w757) -> ()
                    n234 = local write "Total Delta C2(pF)"(w757) -> ()
                    n235 = local write "Total Delta C3(pF)"(w757) -> ()
                    n236 = local write "Current EFuse Read back"(w757) -> ()
                    n237 = local write "RB Reg for HD"(w757) -> ()
                    n238 = To Long Integer(number=0.0 ("No of Loops to RP")) -> (32bit integer=w755:i32)
                    n239 = local write "NOM IDD ON (uA)"(w756) -> ()
                    n240 = local write "NOM IDD OFF(uA)"(w756) -> ()
                    n241 = local write "LPs Count"(w755) -> ()
                    n242 = local write "No LPs to RP"(w755) -> ()
                    n243 = local write "VSA_V3"(w758) -> ()
                    n244 = local write "VSA_V1"(w758) -> ()
                    n245 = local write "VSA_V2"(w758) -> ()
                    n246 = local write "VPI C1"(w758) -> ()
                    n247 = local write "VPI C2"(w758) -> ()
                    n248 = local write "VPI C3"(w758) -> ()
                    n249 = local write "% Delta C"(w758) -> ()
                    n250 = local write "40V_3"(w758) -> ()
                    n251 = local write "40V_2"(w758) -> ()
                    n252 = local write "40V_1"(w758) -> ()
                  }
                }
                n253 = call "WSVCAP SHL Host TL RFFE Write - Multiple DUTs - Common Data.vi"("Data Out"=w669, "error in"=w670, "Log (T)"=w695) -> ("error out"=w717:errorcluster)  [unwired: 12 in]
                n254 = call "Delay T4.vi"("milliseconds to wait"=u32 50, "error in (no error)"=w717) -> ("error out"=w676:errorcluster)  [unwired: 9 in]
                n255 = for {
                  tunnel: [w742] -> w726
                  tunnel: [w741] -> w697
                  tunnel: w695 -> [w740]
                  tunnel: w683 -> [w739]
                  tunnel: w676 -> [w735]
                  tunnel: string[] ["0702013B3B3B", "070201000000"] -> [w731] mode=indexing
                  tunnel: [w730] -> w679 mode=indexing
                  n256 = call "WSVCAP SHL Host TL RFFE Write - Multiple DUTs - Common Data.vi"("Data Out"=w731, "error in"=w735, "Log (T)"=w740) -> ("error out"=w736:errorcluster)  [unwired: 12 in]
                  n257 = local read "IDD Brd(uA)"() -> (w732:string)
                  n258 = call "Delay T4.vi"("milliseconds to wait"=u32 100, "error in (no error)"=w736) -> ("error out"=w737:errorcluster)  [unwired: 9 in]
                  n259 = call "Ke2000 Single Reading.vi"("error in (no error)"=w737, "VISA resource name"=w739) -> ("error out"=w734:errorcluster, "VISA resource name out"=w742:refnum<visa-resource-name>, "uA"=w733:string)  [unwired: 5 in, 2 out]
                  n260 = call "Substration.vi"("error in (no error)"=w734, "Input2"=w732, "Input1"=w733) -> ("error out"=w741:errorcluster, "In1 - In2"=w730:string)  [unwired: 7 in]
                }
                n261 = Index Array(array=w679, index=1) -> (element=w678:string)
                n262 = Index Array(array=w679, index=0) -> (element=w681:string)
                n263 = local read "Clock Rate (Hz)"() -> (w718:dbl)
                n264 = call "Multi Dut Cmd_Header Setting.vi"("WS1050/51"="WS1050/51", "Cmin/Act"="Cmin/Act", "Test Seq"="Test Sequences", "error in (no error)"=w693) -> ("Name 1"=w691:string[], "Name 2"=w690:string[], "Name Header"=w688:string[], "Name 3"=w689:string[], "Cmd 3"=w685:string[], "Cmd 1"=w687:string[], "Cmd 2"=w686:string[], "error out"=w694:errorcluster)  [unwired: 2 in, 2 out]
                "Loops Run" <- w665
              }
              frame #1 {
                w1002 = FALSE ("Log (T)")
                n265 = call "WSVCAP SHL Host TL RFFE Configure.vi"("RFFE Slave Address"=w1013, "Clock Rate (Hz)"=w1011, "error in"=w1003) -> ("Actual Rate (Hz)"=w1023:dbl, "error out"=w1009:errorcluster)  [unwired: 11 in]
                n266 = local write "AR  Measurent(Hz)"(w1023) -> ()
                n267 = Array Size(array=w1014) -> (size(s)=w1026:i32)
                n268 = case shown="2" w996 {
                  tunnel: w1026 -> [w1035 w1067 w1099]
                  tunnel: w1020 -> [w1034 w1066 w1098]
                  tunnel: [w1033 w1065 w1097] -> w1016
                  tunnel: w1015 -> [w1032 w1064 w1096]
                  tunnel: w1014 -> [w1031 w1063 w1095]
                  tunnel: w1009 -> [w1030 w1062 w1094]
                  tunnel: [w1029 w1061 w1093] -> w1008
                  tunnel: w1002 -> [w1028 w1060 w1092]
                  tunnel: [w1027 w1059 w1091] -> w997
                  frame 0, Default {
                    n269 = for {
                      N: w1035 -> [_]
                      tunnel: w1032 -> [w1054]
                      tunnel: w1034 -> [w1052]
                      tunnel: [w1051] -> w1033
                      tunnel: [w1047] -> w1027 mode=indexing
                      tunnel: w1031 -> [w1049]
                      tunnel: w1030 -> [w1037]
                      tunnel: [w1039] -> w1029
                      tunnel: w1028 -> [w1038]
                      i -> [w1046]
                      stop <- w1051 stop-if-true
                      n270 = Index Array(array=w1054, index=w1046) -> (element=w1050:string)
                      n271 = Index Array(array=w1049, index=w1046) -> (element=w1048:string)
                      n272 = local write "STATUS"(w1048) -> ()
                      n273 = call "WSVCAP SHL Host TL RFFE Write - Multiple DUTs - Common Data.vi"("Data Out"=w1050, "error in"=w1037, "Log (T)"=FALSE) -> ("error out"=w1041:errorcluster)  [unwired: 12 in]
                      n274 = call "Delay T4.vi"("milliseconds to wait"=u32 10, "error in (no error)"=w1041) -> ("error out"=w1045:errorcluster)  [unwired: 9 in]
                      n275 = call "WS1050 AD7747 READ 36 DUT.vi"("error in"=w1045, "Log (T)"=w1038, "DUT Mask Mode (All)"=WSVCAP_SHL_I2C_DUT_Mask_Mode_Enum."C1") -> ("error out"=w1043:errorcluster, "AD7747 Values"=w1044:string[][])  [unwired: 7 in]
                      n276 = for {
                        tunnel: w1044 -> [w1057] mode=indexing
                        tunnel: w1043 -> [w1058]
                        tunnel: [w1058] -> w1039
                        tunnel: [w1055] -> w1047 mode=indexing
                        n277 = Index Array(array=w1057, index=1) -> (element=w1055:string)
                      }
                      n278 = Unbundle By Name(w1039) -> ("status"=w1053:bool)
                      n279 = Or(x=w1053, y=w1052) -> (x .or. y?=w1051:bool)
                    }
                  }
                  frame 1 {
                    n280 = for {
                      N: w1067 -> [_]
                      tunnel: w1064 -> [w1086]
                      tunnel: w1066 -> [w1084]
                      tunnel: [w1083] -> w1065
                      tunnel: [w1079] -> w1059 mode=indexing
                      tunnel: w1063 -> [w1081]
                      tunnel: w1062 -> [w1069]
                      tunnel: [w1071] -> w1061
                      tunnel: w1060 -> [w1070]
                      i -> [w1078]
                      stop <- w1083 stop-if-true
                      n281 = Index Array(array=w1086, index=w1078) -> (element=w1082:string)
                      n282 = Index Array(array=w1081, index=w1078) -> (element=w1080:string)
                      n283 = local write "STATUS"(w1080) -> ()
                      n284 = call "WSVCAP SHL Host TL RFFE Write - Multiple DUTs - Common Data.vi"("Data Out"=w1082, "error in"=w1069, "Log (T)"=FALSE) -> ("error out"=w1073:errorcluster)  [unwired: 12 in]
                      n285 = call "Delay T4.vi"("milliseconds to wait"=u32 10, "error in (no error)"=w1073) -> ("error out"=w1077:errorcluster)  [unwired: 9 in]
                      n286 = call "WS1050 AD7747 READ 36 DUT.vi"("error in"=w1077, "Log (T)"=w1070, "DUT Mask Mode (All)"=WSVCAP_SHL_I2C_DUT_Mask_Mode_Enum."C2") -> ("error out"=w1075:errorcluster, "AD7747 Values"=w1076:string[][])  [unwired: 7 in]
                      n287 = for {
                        tunnel: w1076 -> [w1089] mode=indexing
                        tunnel: w1075 -> [w1090]
                        tunnel: [w1090] -> w1071
                        tunnel: [w1087] -> w1079 mode=indexing
                        n288 = Index Array(array=w1089, index=3) -> (element=w1087:string)
                      }
                      n289 = Unbundle By Name(w1071) -> ("status"=w1085:bool)
                      n290 = Or(x=w1085, y=w1084) -> (x .or. y?=w1083:bool)
                    }
                  }
                  frame 2 {
                    n291 = for {
                      N: w1099 -> [_]
                      tunnel: w1096 -> [w1118]
                      tunnel: w1098 -> [w1116]
                      tunnel: [w1115] -> w1097
                      tunnel: [w1111] -> w1091 mode=indexing
                      tunnel: w1095 -> [w1113]
                      tunnel: w1094 -> [w1101]
                      tunnel: [w1103] -> w1093
                      tunnel: w1092 -> [w1102]
                      i -> [w1110]
                      stop <- w1115 stop-if-true
                      n292 = Index Array(array=w1118, index=w1110) -> (element=w1114:string)
                      n293 = Index Array(array=w1113, index=w1110) -> (element=w1112:string)
                      n294 = local write "STATUS"(w1112) -> ()
                      n295 = call "WSVCAP SHL Host TL RFFE Write - Multiple DUTs - Common Data.vi"("Data Out"=w1114, "error in"=w1101, "Log (T)"=FALSE) -> ("error out"=w1105:errorcluster)  [unwired: 12 in]
                      n296 = call "Delay T4.vi"("milliseconds to wait"=u32 10, "error in (no error)"=w1105) -> ("error out"=w1109:errorcluster)  [unwired: 9 in]
                      n297 = call "WS1050 AD7747 READ 36 DUT.vi"("error in"=w1109, "Log (T)"=w1102, "DUT Mask Mode (All)"=WSVCAP_SHL_I2C_DUT_Mask_Mode_Enum."C3") -> ("error out"=w1107:errorcluster, "AD7747 Values"=w1108:string[][])  [unwired: 7 in]
                      n298 = for {
                        tunnel: w1108 -> [w1121] mode=indexing
                        tunnel: w1107 -> [w1122]
                        tunnel: [w1122] -> w1103
                        tunnel: [w1119] -> w1111 mode=indexing
                        n299 = Index Array(array=w1121, index=5) -> (element=w1119:string)
                      }
                      n300 = Unbundle By Name(w1103) -> ("status"=w1117:bool)
                      n301 = Or(x=w1117, y=w1116) -> (x .or. y?=w1115:bool)
                    }
                  }
                }
                n302 = Transpose 2D Array(2D array=w997) -> (transposed array=w1007:string[][])
                "40V_1" <- w1007
                "NOM IDD ON (uA)" <- w1018
                "NOM IDD OFF(uA)" <- w1017
              }
              frame #2 {
                n303 = Array Size(array=w1142) -> (size(s)=w1143:i32)
                n304 = case shown="0, 2, Default" w1126 {
                  tunnel: w1143 -> [w1160 w1192]
                  tunnel: w1142 -> [w1159 w1191]
                  tunnel: w1141 -> [w1158 w1190]
                  tunnel: w1140 -> [w1157 w1189]
                  tunnel: [w1156 w1188] -> w1139
                  tunnel: [w1155 w1187] -> w1137
                  tunnel: w1135 -> [w1154 w1186]
                  tunnel: w1129 -> [w1153 w1185]
                  tunnel: [w1152 w1184] -> w1127
                  frame 0, 2, Default {
                    n305 = for {
                      N: w1160 -> [_]
                      tunnel: w1158 -> [w1179]
                      tunnel: w1157 -> [w1177]
                      tunnel: [w1176] -> w1156
                      tunnel: [w1172] -> w1152 mode=indexing
                      tunnel: w1159 -> [w1174]
                      tunnel: w1154 -> [w1162]
                      tunnel: [w1164] -> w1155
                      tunnel: w1153 -> [w1163]
                      i -> [w1171]
                      stop <- w1176 stop-if-true
                      n306 = Index Array(array=w1179, index=w1171) -> (element=w1175:string)
                      n307 = Index Array(array=w1174, index=w1171) -> (element=w1173:string)
                      n308 = call "WSVCAP SHL Host TL RFFE Write - Multiple DUTs - Common Data.vi"("Data Out"=w1175, "error in"=w1162, "Log (T)"=FALSE) -> ("error out"=w1166:errorcluster)  [unwired: 12 in]
                      n309 = local write "STATUS"(w1173) -> ()
                      n310 = call "Delay T4.vi"("milliseconds to wait"=u32 10, "error in (no error)"=w1166) -> ("error out"=w1170:errorcluster)  [unwired: 9 in]
                      n311 = call "WS1050 AD7747 READ 36 DUT.vi"("error in"=w1170, "Log (T)"=w1163, "DUT Mask Mode (All)"=WSVCAP_SHL_I2C_DUT_Mask_Mode_Enum."C2") -> ("error out"=w1168:errorcluster, "AD7747 Values"=w1169:string[][])  [unwired: 7 in]
                      n312 = for {
                        tunnel: w1169 -> [w1182] mode=indexing
                        tunnel: w1168 -> [w1183]
                        tunnel: [w1183] -> w1164
                        tunnel: [w1180] -> w1172 mode=indexing
                        n313 = Index Array(array=w1182, index=3) -> (element=w1180:string)
                      }
                      n314 = Unbundle By Name(w1164) -> ("status"=w1178:bool)
                      n315 = Or(x=w1178, y=w1177) -> (x .or. y?=w1176:bool)
                    }
                  }
                  frame 1 {
                    n316 = for {
                      N: w1192 -> [_]
                      tunnel: w1190 -> [w1211]
                      tunnel: w1189 -> [w1209]
                      tunnel: [w1208] -> w1188
                      tunnel: [w1204] -> w1184 mode=indexing
                      tunnel: w1191 -> [w1206]
                      tunnel: w1186 -> [w1194]
                      tunnel: [w1196] -> w1187
                      tunnel: w1185 -> [w1195]
                      i -> [w1203]
                      stop <- w1208 stop-if-true
                      n317 = Index Array(array=w1211, index=w1203) -> (element=w1207:string)
                      n318 = Index Array(array=w1206, index=w1203) -> (element=w1205:string)
                      n319 = call "WSVCAP SHL Host TL RFFE Write - Multiple DUTs - Common Data.vi"("Data Out"=w1207, "error in"=w1194, "Log (T)"=FALSE) -> ("error out"=w1198:errorcluster)  [unwired: 12 in]
                      n320 = local write "STATUS"(w1205) -> ()
                      n321 = call "Delay T4.vi"("milliseconds to wait"=u32 10, "error in (no error)"=w1198) -> ("error out"=w1202:errorcluster)  [unwired: 9 in]
                      n322 = call "WS1050 AD7747 READ 36 DUT.vi"("error in"=w1202, "Log (T)"=w1195, "DUT Mask Mode (All)"=WSVCAP_SHL_I2C_DUT_Mask_Mode_Enum."C1") -> ("error out"=w1200:errorcluster, "AD7747 Values"=w1201:string[][])  [unwired: 7 in]
                      n323 = for {
                        tunnel: w1201 -> [w1214] mode=indexing
                        tunnel: w1200 -> [w1215]
                        tunnel: [w1215] -> w1196
                        tunnel: [w1212] -> w1204 mode=indexing
                        n324 = Index Array(array=w1214, index=1) -> (element=w1212:string)
                      }
                      n325 = Unbundle By Name(w1196) -> ("status"=w1210:bool)
                      n326 = Or(x=w1210, y=w1209) -> (x .or. y?=w1208:bool)
                    }
                  }
                }
                n327 = Transpose 2D Array(2D array=w1127) -> (transposed array=w1136:string[][])
                "40V_2" <- w1136
              }
              frame #3 {
                n328 = Array Size(array=w1235) -> (size(s)=w1236:i32)
                n329 = case shown="0, 1, Default" w1220 {
                  tunnel: w1236 -> [w1254 w1286]
                  tunnel: w1235 -> [w1253 w1285]
                  tunnel: w1234 -> [w1252 w1284]
                  tunnel: w1233 -> [w1251 w1283]
                  tunnel: [w1250 w1282] -> w1232
                  tunnel: w1227 -> [w1249 w1281]
                  tunnel: [w1248 w1280] -> w1219
                  tunnel: w1223 -> [w1247 w1279]
                  tunnel: [w1246 w1278] -> w1221
                  frame 0, 1, Default {
                    n330 = for {
                      N: w1254 -> [_]
                      tunnel: w1252 -> [w1273]
                      tunnel: w1251 -> [w1271]
                      tunnel: [w1270] -> w1250
                      tunnel: [w1266] -> w1246 mode=indexing
                      tunnel: w1253 -> [w1268]
                      tunnel: w1249 -> [w1256]
                      tunnel: [w1258] -> w1248
                      tunnel: w1247 -> [w1257]
                      i -> [w1265]
                      stop <- w1270 stop-if-true
                      n331 = Index Array(array=w1273, index=w1265) -> (element=w1269:string)
                      n332 = Index Array(array=w1268, index=w1265) -> (element=w1267:string)
                      n333 = local write "STATUS"(w1267) -> ()
                      n334 = call "WSVCAP SHL Host TL RFFE Write - Multiple DUTs - Common Data.vi"("Data Out"=w1269, "error in"=w1256, "Log (T)"=FALSE) -> ("error out"=w1260:errorcluster)  [unwired: 12 in]
                      n335 = call "Delay T4.vi"("milliseconds to wait"=u32 10, "error in (no error)"=w1260) -> ("error out"=w1264:errorcluster)  [unwired: 9 in]
                      n336 = call "WS1050 AD7747 READ 36 DUT.vi"("error in"=w1264, "Log (T)"=w1257, "DUT Mask Mode (All)"=WSVCAP_SHL_I2C_DUT_Mask_Mode_Enum."C3") -> ("error out"=w1262:errorcluster, "AD7747 Values"=w1263:string[][])  [unwired: 7 in]
                      n337 = for {
                        tunnel: w1263 -> [w1276] mode=indexing
                        tunnel: w1262 -> [w1277]
                        tunnel: [w1277] -> w1258
                        tunnel: [w1274] -> w1266 mode=indexing
                        n338 = Index Array(array=w1276, index=5) -> (element=w1274:string)
                      }
                      n339 = Unbundle By Name(w1258) -> ("status"=w1272:bool)
                      n340 = Or(x=w1272, y=w1271) -> (x .or. y?=w1270:bool)
                    }
                  }
                  frame 2 {
                    n341 = for {
                      N: w1286 -> [_]
                      tunnel: w1284 -> [w1305]
                      tunnel: w1283 -> [w1303]
                      tunnel: [w1302] -> w1282
                      tunnel: [w1298] -> w1278 mode=indexing
                      tunnel: w1285 -> [w1300]
                      tunnel: w1281 -> [w1288]
                      tunnel: [w1290] -> w1280
                      tunnel: w1279 -> [w1289]
                      i -> [w1297]
                      stop <- w1302 stop-if-true
                      n342 = Index Array(array=w1305, index=w1297) -> (element=w1301:string)
                      n343 = Index Array(array=w1300, index=w1297) -> (element=w1299:string)
                      n344 = local write "STATUS"(w1299) -> ()
                      n345 = call "WSVCAP SHL Host TL RFFE Write - Multiple DUTs - Common Data.vi"("Data Out"=w1301, "error in"=w1288, "Log (T)"=FALSE) -> ("error out"=w1292:errorcluster)  [unwired: 12 in]
                      n346 = call "Delay T4.vi"("milliseconds to wait"=u32 10, "error in (no error)"=w1292) -> ("error out"=w1296:errorcluster)  [unwired: 9 in]
                      n347 = call "WS1050 AD7747 READ 36 DUT.vi"("error in"=w1296, "Log (T)"=w1289, "DUT Mask Mode (All)"=WSVCAP_SHL_I2C_DUT_Mask_Mode_Enum."C1") -> ("error out"=w1294:errorcluster, "AD7747 Values"=w1295:string[][])  [unwired: 7 in]
                      n348 = for {
                        tunnel: w1295 -> [w1308] mode=indexing
                        tunnel: w1294 -> [w1309]
                        tunnel: [w1309] -> w1290
                        tunnel: [w1306] -> w1298 mode=indexing
                        n349 = Index Array(array=w1308, index=1) -> (element=w1306:string)
                      }
                      n350 = Unbundle By Name(w1290) -> ("status"=w1304:bool)
                      n351 = Or(x=w1304, y=w1303) -> (x .or. y?=w1302:bool)
                    }
                  }
                }
                n352 = Transpose 2D Array(2D array=w1221) -> (transposed array=w1228:string[][])
                "40V_3" <- w1228
              }
              frame #4 {
                # "VPI Testing @ 35V"
                n353 = call "WS1050 Delta C Calculation.vi"("error in (no error)"=w1351, "DCap Target(pF)"=w1350, "Input"=w1353) -> ("error out"=w1348:errorcluster, "Total Bank Delta C(pF)"=w1341:string[], "% Bank DeltaC"=w1345:string[])  [unwired: 4 in, 2 out]
                n354 = call "WS1050 Delta C Calculation.vi"("error in (no error)"=w1351, "DCap Target(pF)"=w1350, "Input"=w1352) -> ("error out"=w1349:errorcluster, "Total Bank Delta C(pF)"=w1340:string[], "% Bank DeltaC"=w1343:string[])  [unwired: 4 in, 2 out]
                n355 = call "WS1050 Delta C Calculation.vi"("error in (no error)"=w1351, "DCap Target(pF)"=w1350, "Input"=w1344) -> ("error out"=w1347:errorcluster, "Total Bank Delta C(pF)"=w1339:string[], "% Bank DeltaC"=w1342:string[])  [unwired: 4 in, 2 out]
                n356 = Merge Errors(w1348, w1349, w1347) -> (w1346:errorcluster)
                n357 = case shown="1, Default" w1354 {
                  tunnel: w1346 -> [w1384 w1392]
                  tunnel: [w1384 w1392] -> w1313
                  tunnel: w1345 -> [w1380 w1388]
                  tunnel: w1343 -> [w1379 w1387]
                  tunnel: w1342 -> [w1378 w1386]
                  tunnel: w1341 -> [w1383 w1391]
                  tunnel: [w1383 w1391] -> w1338
                  tunnel: w1340 -> [w1382 w1390]
                  tunnel: [w1382 w1390] -> w1337
                  tunnel: w1339 -> [w1381 w1389]
                  tunnel: [w1381 w1389] -> w1336
                  frame 0 {
                    n358 = Build Array(w1380, w1379, w1378) -> (→"% Delta C_T0":string[][])
                  }
                  frame 1, Default {
                    n359 = Build Array(w1388, w1387, w1386) -> (→"% Delta C":string[][])
                  }
                }
                "Total Delta C1(pF)" <- w1338
                "Total Delta C2(pF)" <- w1337
                "Total Delta C3(pF)" <- w1336
                n360 = call "WS1050_51 VPI Header.vi"("VPI Name"="VPI Name", "VPI_Cmd"="VPI_Cmd", "Cmin/Act"=w1311, "WS1050/51"=w1322, "error in (no error)"=w1323) -> ("VPI_1"=w1321:string[], "VPI_2"=w1319:string[], "VPI Header"=w1320:string[], "VPI_3"=w1318:string[], "Cmd_3"=w1315:string[], "Cmd_1"=w1317:string[], "Cmd_2"=w1316:string[], "error out"=w1314:errorcluster)  [unwired: 3 in]
                n361 = Merge Errors(w1314, w1313) -> (w1312:errorcluster)
                n362 = case shown="False" w1328 {
                  tunnel: w1368 -> [w1399 w1437]
                  tunnel: [w1395 w1415] -> w1332
                  tunnel: [w1393 w1439] -> w1367
                  tunnel: [w1393 w1423] -> w1366
                  tunnel: [w1399 w1421] -> w1364
                  tunnel: w1361 -> [w1401 w1438]
                  tunnel: [w1401 w1438] -> w1360
                  tunnel: w1317 -> [_ w1436]
                  tunnel: w1316 -> [_ w1430]
                  tunnel: w1315 -> [_ w1425]
                  tunnel: [w1393 w1435] -> w1357
                  tunnel: w1321 -> [w1398 w1433]
                  tunnel: w1319 -> [_ w1431]
                  tunnel: w1318 -> [_ w1426]
                  tunnel: ["" ("string") w1420] -> w1334
                  tunnel: w1312 -> [w1396 w1412]
                  frame False {
                    n363 = Array Size(array=w1398) -> (size(s)=w1397:i32)
                    n364 = for {
                      N: w1397 -> [_]
                      tunnel: [w1403] -> w1394 mode=indexing
                      shift-right: [w1402] -> w1395
                      shift-left: w1396 -> [w1402]
                      n365 = for {
                        N: 36 -> [_]
                        tunnel: [""] -> w1403 mode=indexing
                      }
                    }
                    n366 = Transpose 2D Array(2D array=w1394) -> (transposed array=w1393:string[][])
                    n367 = local write "VPI C1"(w1393) -> ()
                    n368 = local write "VPI C2"(w1393) -> ()
                    n369 = local write "VPI C3"(w1393) -> ()
                  }
                  frame True {
                    w1414 = FALSE ("Log (T)")
                    # "Set CP to 35V"
                    n370 = call "WSVCAP SHL Host TL RFFE Write - Multiple DUTs - Common Data.vi"("Data Out"="074820", "error in"=w1412, "Log (T)"=w1414) -> ("error out"=w1410:errorcluster)  [unwired: 12 in]
                    n371 = call "Delay T4.vi"("milliseconds to wait"=u32 10, "error in (no error)"=w1410) -> ("error out"=w1416:errorcluster)  [unwired: 9 in]
                    n372 = case shown="3" "CP VPI" {
                      selector: "CP VPI" -> [w1444 w1449 w1454 w1458]
                      tunnel: string[] ["07476F", "074776", "074765", "074769", "07477B"] -> [w1445 w1450 w1455 w1460]
                      tunnel: [w1443 w1448 w1453 w1459] -> w1408
                      tunnel: [w1441 w1446 w1451 w1456] -> w1407
                      tunnel: ["35" ("string") "27.5" ("string") "30.5" ("string") "40.25" ("string")] -> w1420
                      tunnel: w1416 -> [w1441 w1446 w1451 w1456]
                      frame 0, Default {
                        n373 = Index Array(array=w1445, index=w1444) -> (element=w1443:string)
                      }
                      frame 2 {
                        n374 = Index Array(array=w1450, index=w1449) -> (element=w1448:string)
                      }
                      frame 3 {
                        n375 = Index Array(array=w1455, index=w1454) -> (element=w1453:string)
                      }
                      frame 1 {
                        n376 = Index Array(array=w1460, index=w1458) -> (element=w1459:string)
                      }
                    }
                    n377 = Array Size(array=w1433) -> (size(s)=w1440:i32)
                    n378 = call "WSVCAP SHL Host TL RFFE Write - Multiple DUTs - Common Data.vi"("Data Out"=w1408, "error in"=w1407, "Log (T)"=w1414) -> ("error out"=w1419:errorcluster)  [unwired: 12 in]
                    n379 = for {
                      N: w1440 -> [_]
                      tunnel: w1436 -> [w1525]
                      tunnel: w1437 -> [w1523]
                      tunnel: [w1522] -> w1429
                      tunnel: [w1520] -> w1434 mode=indexing
                      tunnel: w1433 -> [w1519]
                      tunnel: w1419 -> [w1508]
                      tunnel: [w1510] -> w1418
                      i -> [w1518]
                      stop <- w1522 stop-if-true
                      n380 = Index Array(array=w1525, index=w1518) -> (element=w1521:string)
                      n381 = Index Array(array=w1519, index=w1518) -> (element=w1517:string)
                      n382 = local write "STATUS"(w1517) -> ()
                      n383 = call "WSVCAP SHL Host TL RFFE Write - Multiple DUTs - Common Data.vi"("Data Out"=w1521, "error in"=w1508, "Log (T)"=FALSE) -> ("error out"=w1516:errorcluster)  [unwired: 12 in]
                      n384 = call "Delay T4.vi"("milliseconds to wait"=u32 10, "error in (no error)"=w1516) -> ("error out"=w1512:errorcluster)  [unwired: 9 in]
                      n385 = call "WS1050 AD7747 READ 36 DUT.vi"("error in"=w1512, "Log (T)"=FALSE, "DUT Mask Mode (All)"=WSVCAP_SHL_I2C_DUT_Mask_Mode_Enum."C1") -> ("error out"=w1514:errorcluster, "AD7747 Values"=w1513:string[][])  [unwired: 7 in]
                      n386 = for {
                        tunnel: [w1528] -> w1520 mode=indexing
                        tunnel: w1514 -> [w1527]
                        tunnel: [w1527] -> w1510
                        tunnel: w1513 -> [w1526] mode=indexing
                        n387 = Index Array(array=w1526, index=1) -> (element=w1528:string)
                      }
                      n388 = Unbundle By Name(w1510) -> ("status"=w1524:bool)
                      n389 = Or(x=w1524, y=w1523) -> (x .or. y?=w1522:bool)
                    }
                    n390 = Transpose 2D Array(2D array=w1434) -> (transposed array=w1439:string[][])
                    "VPI C1" <- w1439
                    n391 = Array Size(array=w1431) -> (size(s)=w1432:i32)
                    n392 = for {
                      N: w1432 -> [_]
                      tunnel: w1430 -> [w1502]
                      tunnel: w1429 -> [w1500]
                      tunnel: [w1499] -> w1422
                      tunnel: [w1497] -> w1428 mode=indexing
                      tunnel: w1431 -> [w1496]
                      tunnel: w1418 -> [w1485]
                      tunnel: [w1487] -> w1417
                      i -> [w1495]
                      stop <- w1499 stop-if-true
                      n393 = Index Array(array=w1502, index=w1495) -> (element=w1498:string)
                      n394 = Index Array(array=w1496, index=w1495) -> (element=w1494:string)
                      n395 = call "WSVCAP SHL Host TL RFFE Write - Multiple DUTs - Common Data.vi"("Data Out"=w1498, "error in"=w1485, "Log (T)"=FALSE) -> ("error out"=w1493:errorcluster)  [unwired: 12 in]
                      n396 = local write "STATUS"(w1494) -> ()
                      n397 = call "Delay T4.vi"("milliseconds to wait"=u32 10, "error in (no error)"=w1493) -> ("error out"=w1489:errorcluster)  [unwired: 9 in]
                      n398 = call "WS1050 AD7747 READ 36 DUT.vi"("error in"=w1489, "Log (T)"=FALSE, "DUT Mask Mode (All)"=WSVCAP_SHL_I2C_DUT_Mask_Mode_Enum."C2") -> ("error out"=w1491:errorcluster, "AD7747 Values"=w1490:string[][])  [unwired: 7 in]
                      n399 = for {
                        tunnel: [w1505] -> w1497 mode=indexing
                        tunnel: w1491 -> [w1504]
                        tunnel: [w1504] -> w1487
                        tunnel: w1490 -> [w1503] mode=indexing
                        n400 = Index Array(array=w1503, index=3) -> (element=w1505:string)
                      }
                      n401 = Unbundle By Name(w1487) -> ("status"=w1501:bool)
                      n402 = Or(x=w1501, y=w1500) -> (x .or. y?=w1499:bool)
                    }
                    n403 = Transpose 2D Array(2D array=w1428) -> (transposed array=w1435:string[][])
                    "VPI C2" <- w1435
                    n404 = Array Size(array=w1426) -> (size(s)=w1427:i32)
                    n405 = for {
                      N: w1427 -> [_]
                      tunnel: w1425 -> [w1479]
                      tunnel: w1422 -> [w1477]
                      tunnel: [w1476] -> w1421
                      tunnel: [w1474] -> w1424 mode=indexing
                      tunnel: w1426 -> [w1473]
                      tunnel: w1417 -> [w1462]
                      tunnel: [w1464] -> w1415
                      i -> [w1472]
                      stop <- w1476 stop-if-true
                      n406 = Index Array(array=w1479, index=w1472) -> (element=w1475:string)
                      n407 = Index Array(array=w1473, index=w1472) -> (element=w1471:string)
                      n408 = call "WSVCAP SHL Host TL RFFE Write - Multiple DUTs - Common Data.vi"("Data Out"=w1475, "error in"=w1462, "Log (T)"=FALSE) -> ("error out"=w1470:errorcluster)  [unwired: 12 in]
                      n409 = local write "STATUS"(w1471) -> ()
                      n410 = call "Delay T4.vi"("milliseconds to wait"=u32 10, "error in (no error)"=w1470) -> ("error out"=w1466:errorcluster)  [unwired: 9 in]
                      n411 = call "WS1050 AD7747 READ 36 DUT.vi"("error in"=w1466, "Log (T)"=FALSE, "DUT Mask Mode (All)"=WSVCAP_SHL_I2C_DUT_Mask_Mode_Enum."C3") -> ("error out"=w1468:errorcluster, "AD7747 Values"=w1467:string[][])  [unwired: 7 in]
                      n412 = for {
                        tunnel: [w1482] -> w1474 mode=indexing
                        tunnel: w1468 -> [w1481]
                        tunnel: [w1481] -> w1464
                        tunnel: w1467 -> [w1480] mode=indexing
                        n413 = Index Array(array=w1480, index=5) -> (element=w1482:string)
                      }
                      n414 = Unbundle By Name(w1464) -> ("status"=w1478:bool)
                      n415 = Or(x=w1478, y=w1477) -> (x .or. y?=w1476:bool)
                    }
                    n416 = Transpose 2D Array(2D array=w1424) -> (transposed array=w1423:string[][])
                    "VPI C3" <- w1423
                  }
                }
                n417 = Insert Into Array(array=w1356, new element=w1320) -> (w1355:string[])  [unwired: 1 in]
                n418 = case shown="True" w1333 {
                  tunnel: w1332 -> [w1370 w1375]
                  tunnel: [w1371 w1374] -> w1331
                  frame False {
                    n419 = call "WSVCAP SHL Host TL RFFE Write - Multiple DUTs - Common Data.vi"("Data Out"="074820", "error in"=w1370, "Log (T)"=FALSE) -> ("error out"=w1371:errorcluster)  [unwired: 12 in]
                  }
                  frame True {
                    n420 = call "WSVCAP SHL Host TL RFFE Write - Multiple DUTs - Common Data.vi"("Data Out"="074800", "error in"=w1375, "Log (T)"=FALSE) -> ("error out"=w1374:errorcluster)  [unwired: 12 in]
                  }
                }
                n421 = call "Delay T4.vi"("milliseconds to wait"=u32 10, "error in (no error)"=w1331) -> ("error out"=w1330:errorcluster)  [unwired: 9 in]
              }
              frame #5 {
                # "VSA Testing"
                n422 = case shown="False" w1531 {
                  tunnel: w1570 -> [w1582 w1596]
                  tunnel: [w1581 w1595] -> w1544
                  tunnel: [w1586 w1602] -> w1560
                  tunnel: w1561 -> [w1586 w1601]
                  tunnel: [w1583 w1599] -> w1549
                  tunnel: [w1583 w1598] -> w1546
                  tunnel: [w1583 w1597] -> w1543
                  tunnel: [w1584 w1600] -> w1550
                  frame False {
                    n423 = for {
                      tunnel: dbl[] [0.0, 0.0, 0.0] -> [w1591] mode=indexing
                      tunnel: [w1590] -> w1584 mode=indexing
                      tunnel: [w1587] -> w1583 mode=indexing
                      shift-right: [w1588] -> w1581
                      shift-left: w1582 -> [w1588]
                      n424 = Number To Fractional String(number=w1591) -> (F-format string=w1592:string)  [unwired: 3 in]
                      n425 = for {
                        N: 36 -> [_]
                        tunnel: w1592 -> [w1594]
                        tunnel: [w1594] -> w1590 mode=indexing
                        tunnel: [""] -> w1587 mode=indexing
                      }
                    }
                  }
                  frame True {
                    n426 = for {
                      tunnel: "VSA Voltage(V)" -> [w1626] mode=indexing
                      tunnel: [w1630] -> w1602
                      tunnel: w1601 -> [w1628]
                      tunnel: [w1627] -> w1599 mode=indexing
                      tunnel: [w1614] -> w1598 mode=indexing
                      tunnel: [w1623] -> w1600 mode=indexing
                      tunnel: [w1608] -> w1597 mode=indexing
                      tunnel: w1596 -> [w1607]
                      tunnel: [w1606] -> w1595
                      w1605 = FALSE ("Log (T)")
                      w1622 = u16 0 items=["Voltage", "Current"] ("Source Mode  (0: Voltage)")
                      n427 = call "Ke2400 Configure Output.vi"("Source Mode  (0: Voltage)"=w1622, "error in (no error)"=w1607, "Compliance  Level (0.1)"=0.1, "Output Level (0)"=w1626, "VISA resource name"=w1628) -> ("error out"=w1634:errorcluster, "VISA resource name out"=w1632:refnum<visa-resource-name>)  [unwired: 5 in]
                      n428 = call "Ke2400 Enable.vi"("error in (no error)"=w1634, "ON/OFF"=TRUE ("Enable Output (T: Enable)"), "VISA resource name"=w1632) -> ("error out"=w1635:errorcluster, "VISA resource name out"=w1630:refnum<visa-resource-name>)  [unwired: 7 in]
                      n429 = call "Delay T4.vi"("milliseconds to wait"=u32 10, "error in (no error)"=w1635) -> ("error out"=w1621:errorcluster)  [unwired: 9 in]
                      n430 = call "WS1050 AD7747 READ 36 DUT.vi"("error in"=w1621, "Log (T)"=w1605, "DUT Mask Mode (All)"=WSVCAP_SHL_I2C_DUT_Mask_Mode_Enum."C1") -> ("error out"=w1618:errorcluster, "AD7747 Values"=w1620:string[][])  [unwired: 7 in]
                      n431 = for {
                        tunnel: w1620 -> [w1646] mode=indexing
                        tunnel: [w1647] -> w1627 mode=indexing
                        tunnel: w1618 -> [w1645]
                        tunnel: [w1645] -> w1617
                        n432 = Index Array(array=w1646, index=1) -> (element=w1647:string)
                      }
                      n433 = call "WS1050 AD7747 READ 36 DUT.vi"("error in"=w1617, "Log (T)"=w1605, "DUT Mask Mode (All)"=WSVCAP_SHL_I2C_DUT_Mask_Mode_Enum."C2") -> ("error out"=w1615:errorcluster, "AD7747 Values"=w1613:string[][])  [unwired: 7 in]
                      n434 = for {
                        tunnel: w1613 -> [w1641] mode=indexing
                        tunnel: [w1642] -> w1614 mode=indexing
                        tunnel: w1615 -> [w1640]
                        tunnel: [w1640] -> w1612
                        n435 = Index Array(array=w1641, index=3) -> (element=w1642:string)
                      }
                      n436 = Number To Fractional String(number=w1626) -> (F-format string=w1625:string)  [unwired: 3 in]
                      n437 = call "WS1050 AD7747 READ 36 DUT.vi"("error in"=w1612, "Log (T)"=w1605, "DUT Mask Mode (All)"=WSVCAP_SHL_I2C_DUT_Mask_Mode_Enum."C3") -> ("error out"=w1610:errorcluster, "AD7747 Values"=w1609:string[][])  [unwired: 7 in]
                      n438 = for {
                        tunnel: w1609 -> [w1637] mode=indexing
                        tunnel: [w1638] -> w1608 mode=indexing
                        tunnel: w1610 -> [w1636]
                        tunnel: [w1636] -> w1606
                        n439 = Index Array(array=w1637, index=5) -> (element=w1638:string)
                      }
                      n440 = for {
                        N: 36 -> [_]
                        tunnel: w1625 -> [w1644]
                        tunnel: [w1644] -> w1623 mode=indexing
                      }
                    }
                    n441 = local write "STATUS"("VSA Testing...." ("STATUS")) -> ()
                  }
                }
                n442 = Transpose 2D Array(2D array=w1550) -> (transposed array=w1548:string[][])
                n443 = Transpose 2D Array(2D array=w1549) -> (transposed array=w1547:string[][])
                n444 = Transpose 2D Array(2D array=w1546) -> (transposed array=w1545:string[][])
                n445 = Transpose 2D Array(2D array=w1543) -> (transposed array=w1542:string[][])
                n446 = call "WS1050_VSA_Convert_Data.vi"("VSA_C3"=w1542, "error in (no error)"=w1544, "VSA_C2"=w1545, "VSA_C1"=w1547, "Voltage"=w1548) -> ("error out"=w1541:errorcluster, "VSA_V3"=w1538:string[][], "VSA_V2"=w1539:string[][], "VSA_V1"=w1540:string[][])  [unwired: 3 in]
                "VSA_V1" <- w1540
                "VSA_V2" <- w1539
                "VSA_V3" <- w1538
                n447 = case shown="True" w1531 {
                  tunnel: w1560 -> [w1574 w1580]
                  tunnel: [w1574 w1579] -> w1559
                  tunnel: w1541 -> [w1573 w1578]
                  tunnel: [w1573 w1575] -> w1558
                  frame False {
                  }
                  frame True {
                    w1576 = u16 0 items=["Voltage", "Current"] ("Source Mode  (0: Voltage)")
                    n448 = call "Ke2400 Configure Output.vi"("Source Mode  (0: Voltage)"=w1576, "error in (no error)"=w1578, "Output Level (0)"=0.0, "VISA resource name"=w1580) -> ("error out"=w1575:errorcluster, "VISA resource name out"=w1579:refnum<visa-resource-name>)  [unwired: 6 in]
                  }
                }
                n449 = call "Delay T4.vi"("milliseconds to wait"=u32 50, "error in (no error)"=w1558) -> ("error out"=w1557:errorcluster)  [unwired: 9 in]
              }
              frame #6 {
                # "Handshake Check and EFuse Readback"
                n450 = Or(x=w1658, y=w1668) -> (x .or. y?=w1667:bool)
                n451 = Add(x=w1680, y=w1679) -> (x+y=w1666:u64)
                n452 = case shown="False" w1667 {
                  tunnel: w1693 -> [w1706 _]
                  tunnel: w1692 -> [w1705 w1711]
                  tunnel: [w1704 w1711] -> w1691
                  tunnel: w1690 -> [w1703 _]
                  tunnel: w1689 -> [w1702 _]
                  tunnel: w1688 -> [w1701 _]
                  tunnel: [w1697 w1710] -> w1687
                  tunnel: [w1696 w1710] -> w1682
                  tunnel: w1666 -> [w1695 _]
                  tunnel: w1673 -> [w1694 _]
                  frame False {
                    n453 = call "WS1050_36DUT_Handshake Check R1_Record All Regs Ver1.0.vi"("file path (use dialog)"=w1706, "Reg1_Bit Cntrl"="Reg1_Bit Cntrl", "File Name"=w1694, "SN"=w1701, "Loop"=w1695, "error"=w1705, "Lot #"=w1703, "Wafer #"=w1702) -> ("Pass/Fail"=→"EFuse Readback Status":bool[], "EFuse Read back"=w1696:string[], "Status"=w1697:string[], "error out"=w1704:errorcluster)  [unwired: 6 in, 2 out]
                    n454 = case shown="1, Default" w1695 {
                      tunnel: w1696 -> [w1707 w1708]
                      frame 0 {
                        "EFuse RB T0" <- w1707
                      }
                      frame 1, Default {
                        "Current EFuse Read back" <- w1708
                      }
                    }
                    n455 = local write "STATUS"("Hand Shake & EFuse Readback...." ("STATUS")) -> ()
                  }
                  frame True {
                    n456 = for {
                      N: 36 -> [_]
                      tunnel: [""] -> w1710 mode=indexing
                    }
                  }
                }
                n457 = Add(x=w1666, y=w1663) -> (x+y=w1664:u64)
                "TTCompleted" <- w1664
                n458 = Number To Engineering String(4:w1664) -> (0:w1678:string)  [unwired: 3 in]
                n459 = Build Array(w1677, w1675, w1674) -> (w1676:string[])
              }
              frame #7 {
                # "Save Data"
                n460 = Increment(x=w1724) -> (x+1=w1723:i32)
                n461 = local write "STATUS"("Saving Data...." ("STATUS")) -> ()
                n462 = Multiply(x=w1723, y=36) -> (x*y=w1718:i32)
                n463 = Path To String(path=w1728) -> (string=w1727:string)
                n464 = Bundle("Test Program"=w1760, "Comment"=w1759, "Data Out"=w1735, "Data Out"=w1734, "CP Voltage"=w1733, w1732, "Data Out"=w1731, "CP Voltage"=w1730, "string"=w1729, "Freq(Hz)"=w1716, "Board#"=w1714) -> (w1715:T8)  [unwired: 1 in]
                n465 = case shown="True" "Debug" {
                  tunnel: w1718 -> [w1767 w1770]
                  tunnel: [w1767 w1768] -> w1717
                  frame False {
                  }
                  frame True {
                    n466 = Multiply(x=w1770, y="No of Rows\nFrom Spread Sheet") -> (x*y=w1768:i32)
                  }
                }
                n467 = call "WS1050_36 DUT SData Ver1.0.vi"("TMN DC\\CAP Data Log File Path"=w1728, "Lot#"=w1762, "Total Delta C1(pF)"=w1738, "VSA_V1"=w1747, "Wafer#"=w1758, "File Name"=w1721, "Total Delta C2(pF)"=w1737, "error in"=w1765, "TP/Comment"=w1715, "EFuse"=w1752, "Data Output C3"=w1740, "Temperature"=w1744, "VSA_V2"=w1748, "VPI C3"=w1742, "Data Output C1"=w1755, "VPI C2"=w1741, "SN"=w1763, "R/W Status"=w1761, "Cap Header"=w1743, "HD/Cycles Completed"=w1751, "Data Output C2"=w1739, "VSA_V3"=w1746, "Current"=w1754, "VPI C1"=w1753, "Total Delta C3(pF)"=w1736) -> ("error out"=w1764:errorcluster)  [unwired: 2 in]
                n468 = Concatenate Strings(w1727, "\\" ("string"), w1721, "_Multi Socket Data.csv" ("string")) -> (w1726:string)
              }
              frame #8 {
                n469 = case shown="True" "Plot Delta Cmin" {
                  tunnel: w1777 -> [w1790 w1805]
                  tunnel: [w1790 w1801] -> w1776
                  tunnel: w1775 -> [_ w1797]
                  tunnel: w1773 -> [_ w1795]
                  frame False {
                  }
                  frame True {
                    n470 = String To Path(string=w1797) -> (path=w1796:path)
                    n471 = call "Delay T4.vi"("milliseconds to wait"=u32 50, "error in (no error)"=w1805) -> ("error out"=w1804:errorcluster)  [unwired: 9 in]
                    n472 = call "36DUT Plot From Spread Sheet.vi"("Plot"="Plot", "No of Rows"=w1795, "error in (no error)"=w1804, "Bank"="Bank", "file path (dialog if empty)"=w1796) -> ("error out"=w1799:errorcluster, "Delta C_Min Plot"=→"Plot_1":dbl[][])  [unwired: 5 in]
                    n473 = call "36DUT Plot From Spread Sheet.vi"("Plot"="Plot", "No of Rows"=w1795, "error in (no error)"=w1799, "Bank"="Bank 2", "file path (dialog if empty)"=w1796) -> ("error out"=w1800:errorcluster, "Delta C_Min Plot"=→"Plot_2":dbl[][])  [unwired: 5 in]
                    n474 = call "36DUT Plot From Spread Sheet.vi"("Plot"="Plot", "No of Rows"=w1795, "error in (no error)"=w1800, "Bank"="Bank 3", "file path (dialog if empty)"=w1796) -> ("error out"=w1801:errorcluster, "Delta C_Min Plot"=→"Plot_3":dbl[][])  [unwired: 5 in]
                  }
                }
                n475 = Get Date/Time In Seconds() -> (seconds since 1Jan1904=w1783:timestamp)
                n476 = Get Date/Time String(seconds (now)=w1783, want seconds? (F)=TRUE) -> (date string=→"date string":string, time string=→"Previous Time":string)  [unwired: 1 in]
                n477 = local write "RB Reg for HD/Cycle"(string[] []) -> ()
                n478 = Greater Or Equal?(x=w1780, y=w1772) -> (x >= y?=w1787:bool)
                n479 = Greater Or Equal?(x=w1779, y=w1772) -> (x >= y?=w1778:bool)
                "No of HD/Cycle\nCompleted" <- w1780
              }
            }
            n480 = Increment(x=w586) -> (x+1=→"Loop \ncompleted":i32)
            n481 = call "Delay T4.vi"("milliseconds to wait"=u32 10, "error in (no error)"=w480) -> ("error out"=w481:errorcluster)  [unwired: 9 in]
            n482 = Compound Arithmetic op=OR(w654, w557, w582) -> (w595:bool)
          }
          "Total Time" <- w405
          n483 = Increment(x=w403) -> (x+1=→"Run Loops":i32)
          n484 = local write "No of HD/Cycle\nCompleted"(u64 0 ("No of HD/Cycle\nCompleted")) -> ()
          n485 = Unbundle By Name(w395) -> ("status"=w409:bool)
          n486 = Compound Arithmetic op=OR(w409, w401, w400) -> (w391:bool)
        }
        n487 = for {
          tunnel: w287 -> [w1817]
          tunnel: w265 -> [w1816]
          tunnel: w316 -> [w1814] mode=indexing
          tunnel: [w1809] -> w285
          tunnel: [w1813] -> w315
          n488 = call "E3631A_Voltage Controller updated.vi"("VISA resource name"=w1816, "I_VDD(A)"=0.5, "Channel Controller"=w1814, "Voltage 1"=0.0, "Voltage 2"=3.3, "error in (no error)"=w1817, "I_3.3V (A)"=0.5) -> ("VISA resource name out"=w1813:refnum<visa-resource-name>, "error out"=w1810:errorcluster)  [unwired: 7 in]
          n489 = call "Delay T4.vi"("milliseconds to wait"=u32 100, "error in (no error)"=w1810) -> ("error out"=w1809:errorcluster)  [unwired: 9 in]
        }
        n490 = VISA Write(VISA resource name=w306, write buffer="SOUR:FUNC VOLT;VOLT:MODE FIX;RANG 100;LEV 0.0;:SENS:FUNC \"CURR\";CURR:PROT 60E-3;RANG 100E-3;:OUTP ON", error in (no error)=w287) -> (VISA resource name out=w304:refnum<visa-resource-name>, error out=w286:errorcluster)  [unwired: 1 out]
        n491 = Merge Errors(w285, w286) -> (w305:errorcluster)
      }
      frame True {
      }
    }
    n492 = local write "stop During HD/Cycles"(w70) -> ()
    n493 = Wait Until Next ms Multiple(millisecond multiple=u32 100) -> ()  [unwired: 1 out]
    n494 = Unbundle By Name(w71) -> ("status"=w89:bool)
    n495 = Or(x=w89, y=w80) -> (x .or. y?=w88:bool)
    "STATUS" <- "Idle...." ("STATUS")
  }
  "Ke2000 Out" <- w22
  "PS1 Out" <- w21
  n496 = local write "stop During HD/Cycles"(w7) -> ()
  n497 = local write "stop"(w7) -> ()
  n498 = case shown="True" w19 {
    tunnel: [w1834 w1837] -> w2
    tunnel: w13 -> [w1834 w1836]
    frame False {
    }
    frame True {
      n499 = local write "Online"(FALSE ("Online")) -> ()
      n500 = call "WSVCAP SHL Host TL Close.vi"("error in"=w1836) -> ("error out"=w1837:errorcluster)  [unwired: 14 in]
    }
  }
  "error out" <- w2
  n501 = VISA Write(VISA resource name=w14, write buffer="SOUR:FUNC VOLT;VOLT:MODE FIX;RANG 100;LEV 0.0;:SENS:FUNC \"CURR\";CURR:PROT 60E-3;RANG 100E-3;:OUTP OFF", error in (no error)=w13) -> (VISA resource name out=→"VISA resource name out":refnum<visa-resource-name>, error out=→"error out 2":errorcluster)  [unwired: 1 out]
